vi "Micro-PL v10.6.0.vi"() -> ()   [LabVIEW 2010]
uses:
  drivers/Oxford ITC/ITCAPPS.LLB/ITCSetup.ctl
  drivers/Oxford ITC/ITCSUBS.LLB/ITCIO.ctl
  drivers/Oxford ITC/BUSGEN.LLB/OxfordAddress.ctl
  drivers/Oxford ITC/ITCSUBS.LLB/ITCVersion.ctl
  subvi/NPC3SG/TypeDefs/NPC3SG Live Controls.ctl
  subvi/NPC3SG/TypeDefs/NPC3SG Current Values.ctl
  subvi/NPC3SG/TypeDefs/NPC3SG Set Positions.ctl
  subvi/ITC503/TypeDefs/ITC503 Settings.ctl
  subvi/ITC503/TypeDefs/ITC503 Current Values.ctl
  subvi/iHR550/TypeDefs/iHR Current Values.ctl
  subvi/iHR550/TypeDefs/iHR Settings.ctl
  subvi/Mapping/TypeDefs/Mapping Spectra Params.ctl
  <vilib>/Utility/miscctls.llb/LVBoundsTypeDef.ctl
  subvi/Symphony/TypeDefs/Symphony Area Format.ctl
  <vilib>/Utility/miscctls.llb/LVPointTypeDef.ctl
  subvi/Mapping/TypeDefs/Mapping Input Parameters v10.6.0.ctl
  subvi/Global Variables.vi
  <vilib>/Analysis/NI_AALBase.lvlib
panel:
  out "Spectrum Raw PX":dbl[][](array[numeric])
  out "Image Raw":i32[][](array[numeric])
  in  "Wavelength Recalculate":bool
  out "CCD Error":errorcluster
  out "Firmware":string="V1.20 CCD_4000"
  out "CCD Gain Number":i32[](array[numeric])=[10, 11, 12, 13, 8, 2]
  out "CCD ADC Number":i32[](array[numeric])=[0, 1, 2, 3, 4]
  out "JYCCDLib.IJYCCDReqd":refnum<k7>
  out "Spectrum Raw WL":dbl[][](array[numeric])
  out "Mapping State Storage":bool
  out "Drive Copy Target":bool
  in  "CCD Shutter":bool caption="Shutter:"
  out "Measurement Running":bool
  out "ITC Running":bool
  out "Drive Running":bool
  out "CCD Running":bool
  out "Mono Running":bool
  in  "Exit":bool
  out "Mono Status":bool
  out "Drive Status":bool
  out "CCD Status":bool
  out "ITC Status":bool
  in  "Register":enum32{"Devices", "Acquisition / Mapping"}(tab)
  in  "Snapshot Folder":path=path "C:/Users/WET-KORR/Desktop/Screenshots"
  in  "Camera Name":string="HD USB Camera"
  out "CCD Temp Graph":dbl(graph)=-134.538067
  out "CCD IDs":u16(ring) items=["CCD1"]
  out "ITC Current Values":T1 {"ITC503 Gradient" format="%.2f"; "ITC503 Setpoint" min=-273.0 max=300000.0 step=0.0001 format="%.1f"; "ITC503 I" format="%_1f"; "ITC503 P" format="%_1f"; "ITC503 Temperature" min=0.0 max=1645.0 step=1e-05 format="%.2f"; "ITC503 Heater" min=0.0 max=100.0 step=0.01 scale=0.0..100.0}
  in  "ITC Settings":T2={"ITC503 Set Setpoint"=0.0, "ITC503 Set Auto Heater"=TRUE, "ITC503 Set Auto PID"=TRUE, "P"=0.0, "I"=0.0, "D"=0.0} {"D" min=0.0 max=100.0 step=0.1 format="%.1f"; "I" min=0.0 max=100.0 step=0.1 format="%.1f"; "P" min=0.0 max=100.0 step=0.1 format="%.1f"; "ITC503 Set Setpoint" min=-273.0 max=300000.0 step=0.1 format="%.1f"}
  in  "ITC Configure":bool
  in  "ITC Connect":bool
  in  "ITC Selector":u16(ring) caption="Select Device" items=["ITC503s"]
  out "Drive Current Values":T3 {"Drive Z Position" min=-273.0 max=300000.0 step=0.0001 format="%.3f"; "Drive Y Position" min=-273.0 max=300000.0 step=0.0001 format="%.3f"; "Drive X Position" min=-273.0 max=300000.0 step=0.0001 format="%.3f"}
  in  "Drive Connection":refnum<visa-resource-name>="COM5" caption="COM Port"
  in  "Drive Connect":bool
  out "Mono Timing":u32 caption="Mono"
  out "Drive Timing":u32 caption="Drive"
  out "ITC Timing":u32 caption="ITC"
  out "CCD Timing":u32 caption="CCD"
  in  "Mono Force Init":bool=TRUE caption="iHR550 Force Init"
  in  "Mono Connect":bool
  in  "Mono ID":string(combo)="iHR550" caption="Monochromator ID"
  in  "CCD Gain":u16(ring)=1 caption="Gain Mode" items=["High Light", "Best Dynamic Range", "High Sensitivity"]
  in  "Image Mode":bool caption="Image Mode?"
  in  "CCD Names":u16(ring) caption="CCD ID" items=["Symphony II"]
  in  "CCD Connect":bool
  out "CCD Temperature":dbl caption="Temp. (°C)" min=10.0 max=160.0 step=0.1 format="%.1f"
  out "CCD Pixel X":i32=2048 caption="X Pixels"
  out "CCD Pixel Y":i32=512 caption="Y Pixels"
  out "CCD Data Size":i32=2048 caption="Data Size"
  in  "CCD ADC":u16(ring) caption="ADC Frequency" items=["20 kHz       ", " 1 MHz       ", " 1 MHz Ultra ", "500 kHz Wrap"]
  in  "CCD Configure":bool
  in  "CCD Area":T4={"XStart"=1, "YStart"=1, "XStop"=2048, "YStop"=512, "XBin"=1, "YBin"=1}
  in  "Spectrum Axis":u16(ring)=1 caption="Axis" items=["Pixel", "Wavelength", "Energy"]
  in  "Spectrum Autosave":bool caption="iHR550 Force Init"
  in  "CCD Preview":bool
  in  "CCD Acquire":bool
  in  "Spectrum Settings":T5={"Integration Time"=1.0, "Repetitions"=1, "Mapping Spectra"=TRUE} caption="Mapping Spectra Settings" {"Repetitions" min=1 max=100 step=1; "Integration Time" min=0.1 max=6000.0 step=0.1 format="%.1f"}
  in  "CCD Current Rep.":string="0/0"
  out "Spectrum":cluster{dbl[], dbl[]}[](graph)
  in  "Spectrum Noise":i64 caption="Noise Level"
  in  "Spectrum Load":bool
  in  "Spectrum Save":bool
  out "Image":dbl[][](graph)
  in  "Spectrum Maximize":bool
  in  "Video Show":bool
  in  "Drive GoTo":bool caption="Objective Move Abs."
  in  "Drive New Positions":T6 {"Drive X Set" min=10.0 max=160.0 step=0.1 format="%.3f"; "Drive Z Set" min=10.0 max=160.0 step=0.1 format="%.3f"; "Drive Y Set" min=10.0 max=160.0 step=0.1 format="%.3f"}
  out "Drive Live Current Values":T3 {"Drive Z Position" min=-273.0 max=300000.0 step=0.0001 format="%.3f"; "Drive Y Position" min=-273.0 max=300000.0 step=0.0001 format="%.3f"; "Drive X Position" min=-273.0 max=300000.0 step=0.0001 format="%.3f"}
  in  "Drive Live Controls":T7={"Snapshot"=FALSE, "Move Step"=0.5, "Move Home"=FALSE, "Move Down"=FALSE, "Move Up"=FALSE, "Move Left"=FALSE, "Move Right"=FALSE, "Move Out"=FALSE, "Move In"=FALSE} {"Move Step" min=0.0 max=30.0 step=0.1 format="%.3f"}
  in  "Mapping Start":bool
  in  "Mono Configure":bool
  in  "Mono Settings":T8={"iHR550 Set Exit Mirror"=2, "iHR550 Set Side Exit"=0.0, "iHR550 Set Front Entrance"=0.0, "iHR550 Set Wavelength"=897.9988, "iHR550 Set Grating"=0, "iHR550 Set Grating Switch"=FALSE, "iHR550 Set Wavelength Switch"=FALSE, "iHR550 Set Mirror Switch"=FALSE, "iHR550 Set Slits Switch"=FALSE} {"iHR550 Set Grating" items=["1800"=1, "600"=2, "150"=3]; "iHR550 Set Wavelength" min=0.0 max=1500.0 step=1.0; "iHR550 Set Side Exit" min=0.0 max=2000.0 step=1.0; "iHR550 Set Exit Mirror" items=["Front"=2, "Side"=3]}
  out "Mono Current Values":T9={"iHR 550 Front Entrance"=0.0, "iHR550 Side Exit"=0.0, "iHR550 Wavelength"=897.9988, "iHR550 Exit Mirror"=2, "iHR550 Grating"="1", "Grating Index"=1} {"iHR550 Exit Mirror" items=["EntranceMirror", "ExitMirror", "Front", "Side"]}
  out "ITC Temp Storage":dbl
  out "Runtime":u32
  out "ITC Gradient Time":i64
  out "ITC Read":bool
  out "CCD Read":bool
  out "Mono Read":bool
  out "Drive Read":bool
  out "Spectrum Properties":cluster{"Position":T10, "Plot Area Size":T10}={"Position"={"Width"=36, "Height"=367}, "Plot Area Size"={"Width"=496, "Height"=264}}
  in  "Auto Folder":path caption="Ausgewählter Pfad"
  out "Wavelengths (nm)":dbl[](array[numeric])
  out "iHR550 RefNum":refnum<k7> caption="Mono RefNum out"
  out "ITC Setup":T11={"Description"="", "IO Info"={"Address"={"Com Port"=1, "ISOBUS Address"=1, "GPIB Address"=24, "Communication"=enum."ISOBUS"}, "Version"=enum."ITC503", "Ch 1 dec places"=1, "Ch 2 dec places"=1, "Ch 3 dec places"=1, "Ch1 Name"="", "Ch2 Name"="", "Ch3 Name"=""}}
  # "Correlation Setup"
  # "Active"
  # "Active"
  # "ITC"
  # "iHR"
  # "Drive"
  # "CCD"
  # "Status"
  # "CCD"
  # "ITC"
  # "iHR"
  # "Drive"
  # "Video"
  # "Cryostat"
  # "Drives"
  # "Timing"
  # "Monochromator"
  # "CCD"
  # "CCD"
  # "Acquisition"
  # "Drive Control"
  # "XY"
  # "Z"
  # "Mapping"
  # "Launch the Spectral Mapping VI and Raman Tool Set 2.0 in a new window."
  # "Monochromator"
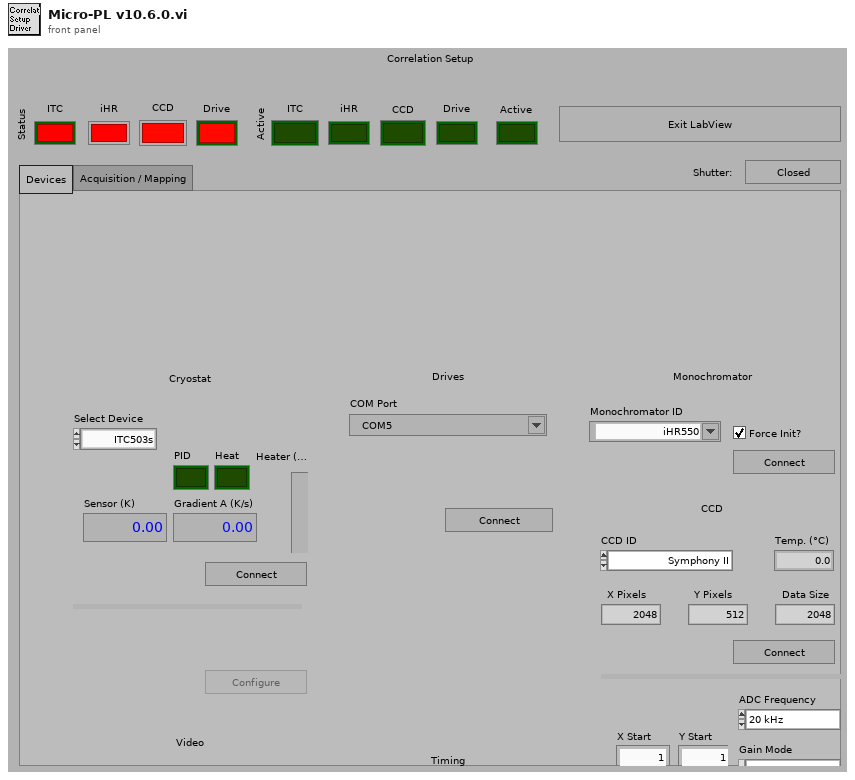
[diagram p1: front panel]
types:
  T1 = typedef "ITC503 Current Values.ctl" = cluster{"ITC503 Heater":dbl, "ITC503 Temperature":dbl, "ITC503 P":dbl, "ITC503 I":dbl, "ITC503 D":dbl, "ITC503 Setpoint":dbl, "ITC503 Gradient":dbl, "ITC503 Heater Auto":bool, "ITC503 PID Auto":bool}
  T2 = typedef "ITC503 Settings.ctl" = cluster{"ITC503 Set Setpoint":dbl, "ITC503 Set Auto Heater":bool, "ITC503 Set Auto PID":bool, "P":dbl, "I":dbl, "D":dbl}
  T3 = typedef "NPC3SG Current Values.ctl" = cluster{"Drive X Position":dbl, "Drive Y Position":dbl, "Drive Z Position":dbl}
  T4 = typedef "Symphony Area Format.ctl" = cluster{"XStart":i32, "YStart":i32, "XStop":i32, "YStop":i32, "XBin":i32, "YBin":i32}
  T5 = typedef "Mapping Spectra Params.ctl" = cluster{"Integration Time":dbl, "Repetitions":u16, "Mapping Spectra":bool}
  T6 = typedef "NPC3SG Set Positions.ctl" = cluster{"Drive X Set":dbl, "Drive Y Set":dbl, "Drive Z Set":dbl}
  T7 = typedef "NPC3SG Live Controls.ctl" = cluster{"Snapshot":bool, "Move Step":dbl, "Move Home":bool, "Move Down":bool, "Move Up":bool, "Move Left":bool, "Move Right":bool, "Move Out":bool, "Move In":bool}
  T8 = typedef "iHR Settings.ctl" = cluster{"iHR550 Set Exit Mirror":u16, "iHR550 Set Side Exit":dbl, "iHR550 Set Front Entrance":dbl, "iHR550 Set Wavelength":dbl, "iHR550 Set Grating":u16, "iHR550 Set Grating Switch":bool, "iHR550 Set Wavelength Switch":bool, "iHR550 Set Mirror Switch":bool, "iHR550 Set Slits Switch":bool}
  T9 = typedef "iHR Current Values.ctl" = cluster{"iHR 550 Front Entrance":dbl, "iHR550 Side Exit":dbl, "iHR550 Wavelength":dbl, "iHR550 Exit Mirror":i32, "iHR550 Grating":string, "Grating Index":i32}
  T10 = typedef "LVBoundsTypeDef.ctl" = cluster{"Width":u32, "Height":u32}
  T11 = typedef "ITCSetup.ctl" = cluster{"Description":string, "IO Info":T12}
  T12 = typedef "ITCIO.ctl" = cluster{"Address":T13, "Version":T14, "Ch 1 dec places":i16, "Ch 2 dec places":i16, "Ch 3 dec places":i16, "Ch1 Name":string, "Ch2 Name":string, "Ch3 Name":string}
  T13 = typedef "OxfordAddress.ctl" = cluster{"Com Port":i32, "ISOBUS Address":i32, "GPIB Address":i16, "Communication":enum16{"RS232", "ISOBUS", "GPIB", "Gateway"}}
  T14 = typedef "ITCVersion.ctl" = enum16{"ITC502", "ITC503", "ITC601"}
  T15 = enum8{"Enabled", "Disabled", "Disabled and Grayed Out"}
  T16 = typedef "LVPointTypeDef.ctl" = cluster{"Horizontal":i16, "Vertical":i16}
  T17 = typedef "Mapping Input Parameters v10.6.0.ctl" = cluster{"Drive Connection Port":refnum<visa-resource-name>, "ITC503 Current Values":T1, "Wavelengths (nm)":dbl[], "Drive Current Values":T3, "iHR Current Values":T9, "Spectra Settings":T5, "CCD3500 Temperature":dbl, "Simulate Drive":bool, "Simulate Spectra":bool, "JYCCDLib.IJYCCDReqd":refnum<k7>, "CCD Area":T4, "CCD Gain":u16, "CCD ADC":u16}
  T18 = cluster{"Intensities":dbl[], "Wavelengths":dbl[]}[]
  T19 = typedef "LVPositionTypeDef.ctl" = cluster{"Left":i32, "Top":i32}
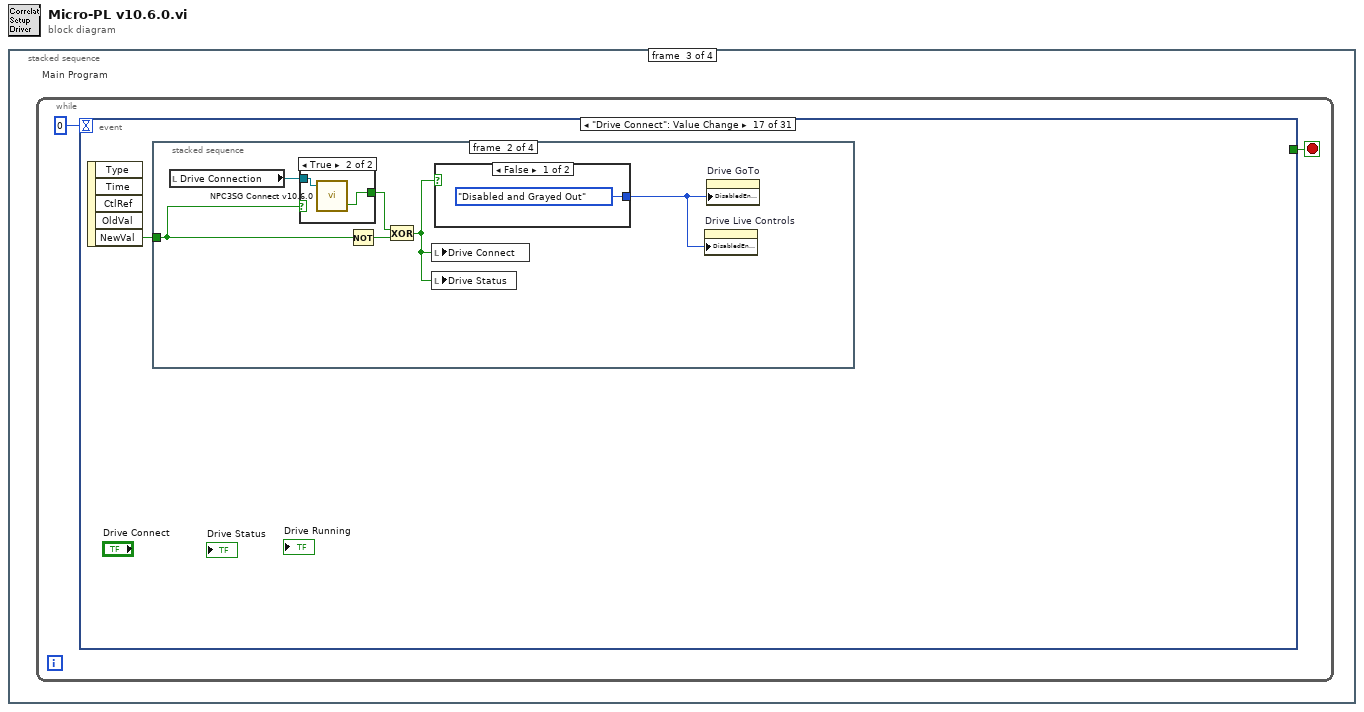
[diagram p0: block diagram]
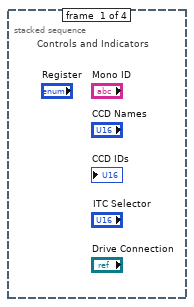
[diagram p2: hidden frame]
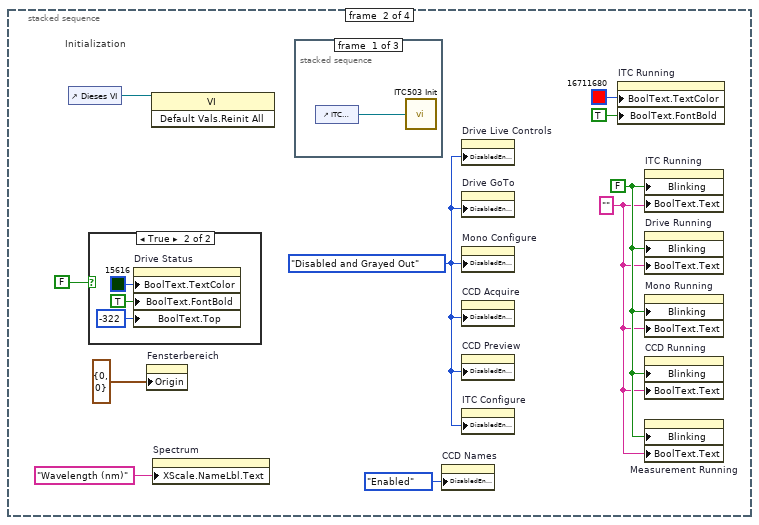
[diagram p3: hidden frame]
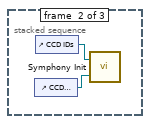
[diagram p4: hidden frame]
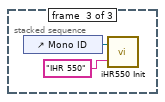
[diagram p5: hidden frame]
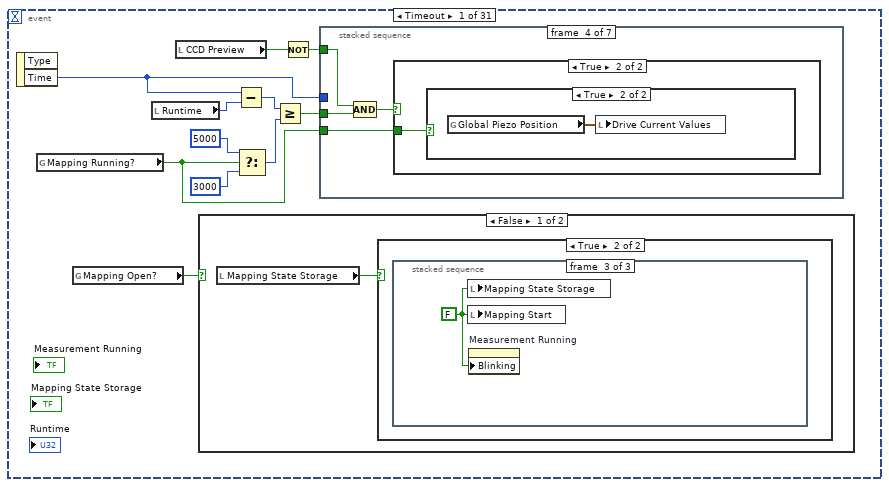
[diagram p7: hidden frame]
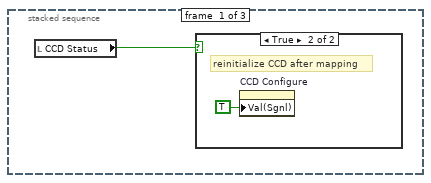
[diagram p9: hidden frame]
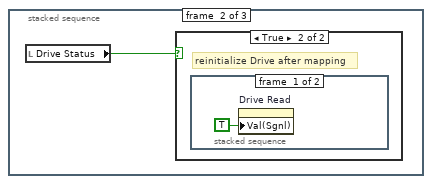
[diagram p11: hidden frame]
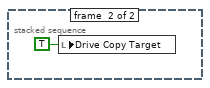
[diagram p13: hidden frame]
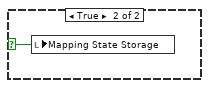
[diagram p14: hidden frame]
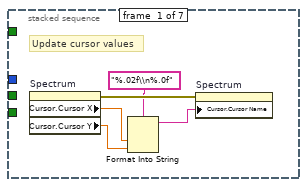
[diagram p15: hidden frame]
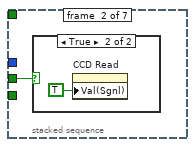
[diagram p16: hidden frame]
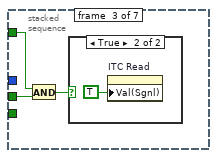
[diagram p18: hidden frame]
diagram:
  n1 = stacked-sequence {
    frame #0 {
      # "Controls and Indicators"
    }
    frame #1 {
      w3 = "" ("Boolean Text.Text")
      w4 = FALSE ("Blinking")
      w7 = T15."Disabled and Grayed Out" ("Deaktiviert")
      # "Initialization"
      n2 = control-ref of="Dieses VI"() -> (w10:refnum<vi>)
      n3 = case shown="True" FALSE {
        frame False {
        }
        frame True {
          n4 = property on="Drive Status" class="Bool (strict)"("BoolText.TextColor"=u32 15616, "BoolText.FontBold"=TRUE ("Boolescher Text.Schriftart:Fett"), "BoolText.Top"=-322 ("Boolescher Text.Position:Oben")) -> ()  [unwired: 2 in, 2 out]
        }
      }
      n5 = property on="Fensterbereich" class="Pane"("Origin"=T16 {"Horizontal"=0, "Vertical"=0}) -> ()  [unwired: 2 in, 2 out]
      n6 = invoke class="VI" method="Default Vals.Reinit All"(reference=w10) -> ()  [unwired: 2 in, 3 out]
      n7 = property on="Spectrum" class="XYGraph (strict)"("XScale.NameLbl.Text"="Wavelength (nm)" ("X Scale.Name Label.Text")) -> ()  [unwired: 2 in, 2 out]
      n8 = stacked-sequence {
        frame #0 {
          n9 = control-ref of="ITC Selector"() -> (w11:refnum<vi>)
          n10 = call "ITC503 Init.vi"("ITC Selector"=w11) -> ()  [unwired: 1 in]
        }
        frame #1 {
          n11 = control-ref of="CCD Names"() -> (w12:refnum<vi>)
          n12 = control-ref of="CCD IDs"() -> (w13:refnum<vi>)
          n13 = call "Symphony Init.vi"("Device Names"=w12, "Device IDs"=w13) -> ()
        }
        frame #2 {
          n14 = control-ref of="Mono ID"() -> (w15:refnum<vi>)
          n15 = call "iHR550 Init.vi"("Mono ID"=w15, "Target ID"="IHR 550") -> ()  [unwired: 1 in]
        }
      }
      n16 = property on="CCD Names" class="Ring (strict)"("DisabledEnum"=T15."Enabled" ("Disabled")) -> ()  [unwired: 2 in, 2 out]
      n17 = property on="Drive Live Controls" class="Clust (strict)"("DisabledEnum"=w7) -> ()  [unwired: 2 in, 2 out]
      n18 = property on="Drive GoTo" class="Bool (strict)"("DisabledEnum"=w7) -> ()  [unwired: 2 in, 2 out]
      n19 = property on="Mono Configure" class="Bool (strict)"("DisabledEnum"=w7) -> ()  [unwired: 2 in, 2 out]
      n20 = property on="CCD Acquire" class="Bool (strict)"("DisabledEnum"=w7) -> ()  [unwired: 2 in, 2 out]
      n21 = property on="CCD Preview" class="Bool (strict)"("DisabledEnum"=w7) -> ()  [unwired: 2 in, 2 out]
      n22 = property on="ITC Configure" class="Bool (strict)"("DisabledEnum"=w7) -> ()  [unwired: 2 in, 2 out]
      n23 = property on="ITC Running" class="Bool (strict)"("BoolText.TextColor"=u32 16711680, "BoolText.FontBold"=TRUE ("Boolean Text.Font:Bold")) -> ()  [unwired: 2 in, 2 out]
      n24 = property on="ITC Running" class="Bool (strict)"("Blinking"=w4, "BoolText.Text"=w3) -> ()  [unwired: 2 in, 2 out]
      n25 = property on="Drive Running" class="Bool (strict)"("Blinking"=w4, "BoolText.Text"=w3) -> ()  [unwired: 2 in, 2 out]
      n26 = property on="Mono Running" class="Bool (strict)"("Blinking"=w4, "BoolText.Text"=w3) -> ()  [unwired: 2 in, 2 out]
      n27 = property on="CCD Running" class="Bool (strict)"("Blinking"=w4, "BoolText.Text"=w3) -> ()  [unwired: 2 in, 2 out]
      n28 = property on="Measurement Running" class="Bool (strict)"("Blinking"=w4, "BoolText.Text"=w3) -> ()  [unwired: 2 in, 2 out]
    }
    frame #2 {
      # "Main Program"
      n29 = while "Main-Program" {
        stop <- w20 stop-if-true
        n30 = event shown="[16] \"Drive Connect\": Value Change" {
          selector: _ -> [_ _ _ _ _ _ _ _ _ _ _ _ _ _ _ _ _ _ _ _ _ _ _ _ _ _ _ _ _ _ _]
          dyn-events: _ -> [_ _ _ _ _ _ _ _ _ _ _ _ _ _ _ _ _ _ _ _ _ _ _ _ _ _ _ _ _ _ _]
          timeout: 0 -> [_ _ _ _ _ _ _ _ _ _ _ _ _ _ _ _ _ _ _ _ _ _ _ _ _ _ _ _ _ _ _]
          tunnel: [_ w69 _ _ _ _ _ _ _ _ _ _ _ _ _ _ _ _ _ _ _ _ _ _ _ _ _ _ _ _ _] -> w20
          event Timeout {
            n31 = event-data() -> ("Time"=w27:u32)  [unwired: 1 in, 1 out]
            n32 = global read "Global Variables.vi" "Mapping Running?"() -> (w22:bool)
            n33 = global read "Global Variables.vi" "Mapping Open?"() -> (w21:bool)
            n34 = local read "Runtime"() -> (w26:u32)
            n35 = local read "CCD Preview"() -> (w29:bool)
            n36 = case shown="False" w21 {
              selector: w21 -> [_ w39]
              frame False {
                n37 = local read "Mapping State Storage"() -> (w32:bool)
                n38 = case shown="True" w32 {
                  frame False {
                  }
                  frame True {
                    n39 = stacked-sequence {
                      frame #0 {
                        n40 = local read "CCD Status"() -> (w33:bool)
                        n41 = case shown="True" w33 {
                          frame False {
                          }
                          frame True {
                            # "reinitialize CCD after mapping"
                            n42 = property on="CCD Configure" class="Bool (strict)"("Val(Sgnl)"=TRUE ("Value (Signaling)")) -> ()  [unwired: 2 in, 2 out]
                          }
                        }
                      }
                      frame #1 {
                        n43 = local read "Drive Status"() -> (w35:bool)
                        n44 = case shown="True" w35 {
                          frame False {
                          }
                          frame True {
                            # "reinitialize Drive after mapping"
                            n45 = stacked-sequence {
                              frame #0 {
                                n46 = property on="Drive Read" class="Bool (strict)"("Val(Sgnl)"=TRUE ("Value (Signaling)")) -> ()  [unwired: 2 in, 2 out]
                              }
                              frame #1 {
                                n47 = local write "Drive Copy Target"(TRUE ("Copy Drive Target")) -> ()
                              }
                            }
                          }
                        }
                      }
                      frame #2 {
                        w38 = FALSE ("Mapping Start")
                        n48 = local write "Mapping State Storage"(w38) -> ()
                        n49 = local write "Mapping Start"(w38) -> ()
                        n50 = property on="Measurement Running" class="Bool (strict)"("Blinking"=w38) -> ()  [unwired: 2 in, 2 out]
                      }
                    }
                  }
                }
              }
              frame True {
                n51 = local write "Mapping State Storage"(w39) -> ()
              }
            }
            n52 = Subtract(x=w27, y=w26) -> (x-y=w30:u32)
            n53 = Select(t=u32 5000 ("y"), s=w22, f=u32 3000 ("y")) -> (s? t:f=w23:u32)
            n54 = Greater Or Equal?(x=w30, y=w23) -> (x >= y?=w31:bool)
            n55 = Not(x=w29) -> (.not. x?=w28:bool)
            n56 = stacked-sequence {
              tunnel: w31 -> [_ w45 w49 w54 w61 _ w66]
              tunnel: w27 -> [_ _ _ _ _ _ w67]
              tunnel: w28 -> [_ _ w48 w53 w60 w63 _]
              tunnel: w22 -> [_ _ _ w51 w58 _ _]
              frame #0 {
                # "Update cursor values"
                n57 = property on="Spectrum" class="XYGraph (strict)"() -> (error out=w44:errorcluster, "Cursor.Cursor X"=w43:dbl, "Cursor.Cursor Y"=w42:dbl)  [unwired: 2 in, 1 out]
                n58 = Format Into String(format string="%.02f\\n%.0f", w43, w42) -> (resulting string=w40:string)  [unwired: 2 in, 1 out]
                n59 = property on="Spectrum" class="XYGraph (strict)"(error in=w44, "Cursor.Cursor Name"=w40) -> ()  [unwired: 1 in, 2 out]
              }
              frame #1 {
                n60 = case shown="True" w45 {
                  frame False {
                  }
                  frame True {
                    n61 = property on="CCD Read" class="Bool (strict)"("Val(Sgnl)"=TRUE ("Value (Signaling)")) -> ()  [unwired: 2 in, 2 out]
                  }
                }
              }
              frame #2 {
                n62 = And(x=w48, y=w49) -> (x .and. y?=w47:bool)
                n63 = case shown="True" w47 {
                  frame False {
                  }
                  frame True {
                    n64 = property on="ITC Read" class="Bool (strict)"("Val(Sgnl)"=TRUE ("Value (Signaling)")) -> ()  [unwired: 2 in, 2 out]
                  }
                }
              }
              frame #3 {
                n65 = Compound Arithmetic op=AND(w53, w54) -> (w52:bool)
                n66 = case shown="True" w52 {
                  tunnel: w51 -> [_ w55]
                  frame False {
                  }
                  frame True {
                    n67 = case shown="True" w55 {
                      frame False {
                        n68 = property on="Drive Read" class="Bool (strict)"("Val(Sgnl)"=TRUE ("Value (Signaling)")) -> ()  [unwired: 2 in, 2 out]
                      }
                      frame True {
                        n69 = global read "Global Variables.vi" "Global Piezo Position"() -> (w57:T3)
                        n70 = local write "Drive Current Values"(w57) -> ()
                      }
                    }
                  }
                }
              }
              frame #4 {
                n71 = Compound Arithmetic op=AND(w60, w61, w58) -> (w59:bool)
                n72 = case shown="True" w59 {
                  frame False {
                  }
                  frame True {
                    n73 = property on="Mono Read" class="Bool (strict)"("Val(Sgnl)"=TRUE ("Value (Signaling)")) -> ()  [unwired: 2 in, 2 out]
                  }
                }
              }
              frame #5 {
                n74 = case shown="False" w63 {
                  frame False {
                    n75 = flat-sequence {
                      frame #0 {
                        w64 = u32 50  # CCD buffer
                        n76 = Wait (ms)(milliseconds to wait=w64) -> ()  [unwired: 1 out]
                      }
                      frame #1 {
                        n77 = property on="CCD Acquire" class="Bool (strict)"("Val(Sgnl)"=TRUE ("Wert (signalisierend)")) -> ()  [unwired: 2 in, 2 out]
                      }
                    }
                  }
                  frame True {
                  }
                }
              }
              frame #6 {
                # "Set runtime counter"
                n78 = case shown="True" w66 {
                  tunnel: w67 -> [_ w68]
                  frame False {
                  }
                  frame True {
                    n79 = local write "Runtime"(w68) -> ()
                  }
                }
              }
            }
          }
          event "Exit": Value Change {
            n80 = event-data() -> ("NewVal"=w69:bool)  [unwired: 1 in, 4 out]
            n81 = stacked-sequence {
              frame #0 {
                n82 = local read "CCD Status"() -> (w70:bool)
                n83 = case shown="True" w70 {
                  frame False {
                  }
                  frame True {
                    n84 = local read "JYCCDLib.IJYCCDReqd"() -> (w71:refnum<k7>)
                    n85 = Close Reference(reference=w71) -> ()  [unwired: 1 in, 1 out]
                  }
                }
              }
              frame #1 {
                n86 = local read "Drive Status"() -> (w72:bool)
                n87 = case shown="True" w72 {
                  frame False {
                  }
                  frame True {
                    n88 = local read "Drive Connection"() -> (w73:refnum<visa-resource-name>)
                    n89 = call "NPC3SG Close.vi"("Drive Visa Name"=w73) -> ()  [unwired: 4 in]
                  }
                }
              }
            }
          }
          event "Mono Connect": Value Change {
            n90 = event-data() -> ("NewVal"=w74:bool)  [unwired: 1 in, 4 out]
            n91 = stacked-sequence {
              tunnel: w74 -> [_ w77 _]
              frame #0 {
                n92 = property on="Mono Running" class="Bool (strict)"("Blinking"=TRUE ("Blinkend")) -> ()  [unwired: 2 in, 2 out]
              }
              frame #1 {
                n93 = case shown="False" w77 {
                  selector: w77 -> [w81 _]
                  tunnel: [w81 w93] -> w76
                  frame False {
                    # "disconnect"
                  }
                  frame True {
                    # "connect"
                    n94 = local read "Mono Force Init"() -> (w91:bool)
                    n95 = control-ref of="iHR550 Set Grating"() -> (w92:refnum<vi>)
                    n96 = local read "Mono ID"() -> (w94:string)
                    n97 = call "iHR550 Connect.vi"("Force\nInitialization"=w91, "Grating Selector"=w92, "Mono ID"=w94) -> ("Initialized"=w93:bool, "iHR550 RefNum"=w90:refnum<k7>)  [unwired: 2 in, 4 out]
                    n98 = local write "iHR550 RefNum"(w90) -> ()
                    n99 = call "iHR550 Read Values v10.5.0.vi"("JYMONOLib.IJYMonoReqd"=w90) -> ("iHR Current Values"=w82:T9)  [unwired: 1 in]
                    n100 = Unbundle By Name(w82) -> ("iHR 550 Front Entrance"=w88:dbl, "iHR550 Side Exit"=w87:dbl, "iHR550 Wavelength"=w86:dbl, "iHR550 Exit Mirror"=w85:i32, "Grating Index"=w83:i32)
                    n101 = local write "Mono Current Values"(w82) -> ()
                    n102 = Bundle By Name(cluster=T8 {"iHR550 Set Exit Mirror"=0, "iHR550 Set Side Exit"=0.0, "iHR550 Set Front Entrance"=0.0, "iHR550 Set Wavelength"=0.0, "iHR550 Set Grating"=0, "iHR550 Set Grating Switch"=FALSE, "iHR550 Set Wavelength Switch"=FALSE, "iHR550 Set Mirror Switch"=FALSE, "iHR550 Set Slits Switch"=FALSE} ("iHR Settings"), "iHR550 Set Front Entrance"=w88, "iHR550 Set Side Exit"=w87, "iHR550 Set Wavelength"=w86, "iHR550 Set Exit Mirror"=w85, "iHR550 Set Grating"=w83) -> (w84:T8)
                    n103 = local write "Mono Settings"(w84) -> ()
                  }
                }
                n104 = case shown="False" w76 {
                  tunnel: [T15."Disabled and Grayed Out" ("Deaktiviert") T15."Enabled" ("Deaktiviert")] -> w78
                  frame False {
                  }
                  frame True {
                  }
                }
                n105 = local write "Mono Connect"(w76) -> ()
                n106 = local write "Mono Status"(w76) -> ()
                n107 = property on="Mono Configure" class="Bool (strict)"("DisabledEnum"=w78) -> ()  [unwired: 2 in, 2 out]
              }
              frame #2 {
                w96 = TRUE ("Wert (signalisierend)")
                w95 = FALSE ("Blinkend")
                n108 = local write "Mono Force Init"(w95) -> ()
                n109 = property on="Mono Running" class="Bool (strict)"("Blinking"=w95) -> ()  [unwired: 2 in, 2 out]
                n110 = property on="Mono Read" class="Bool (strict)"("Val(Sgnl)"=w96) -> ()  [unwired: 2 in, 2 out]
                n111 = property on="Wavelength Recalculate" class="Bool (strict)"("Val(Sgnl)"=w96) -> ()  [unwired: 2 in, 2 out]
              }
            }
          }
          event "Mono Read": Value Change {
            n112 = event-data() -> ("NewVal"=w100:bool)  [unwired: 1 in, 4 out]
            n113 = local read "Mono Status"() -> (w99:bool)
            n114 = And(x=w99, y=w100) -> (x .and. y?=w98:bool)
            n115 = case shown="False" w98 {
              tunnel: [u32 0 w102] -> w97
              frame False {
              }
              frame True {
                n116 = stacked-sequence {
                  seq-local: [w103 _ _] -> [_ _ w106]
                  tunnel: [_ _ w107] -> w102
                  frame #0 {
                    n117 = Tick Count (ms)() -> (millisecond timer value=w103:u32)
                  }
                  frame #1 {
                    n118 = local read "iHR550 RefNum"() -> (w105:refnum<k7>)
                    n119 = call "iHR550 Read Values v10.5.0.vi"("JYMONOLib.IJYMonoReqd"=w105) -> ("iHR Current Values"=w104:T9)  [unwired: 1 in]
                    n120 = local write "Mono Current Values"(w104) -> ()
                    n121 = global write "Global Variables.vi" "Global iHR Values"(w104) -> ()
                  }
                  frame #2 {
                    n122 = Tick Count (ms)() -> (millisecond timer value=w108:u32)
                    n123 = Subtract(x=w108, y=w106) -> (x-y=w107:u32)
                  }
                }
              }
            }
            "Mono Timing" <- w97
          }
          event "Mono Configure": Value Change {
            n124 = event-data() -> ("NewVal"=w109:bool)  [unwired: 1 in, 4 out]
            n125 = stacked-sequence {
              tunnel: w109 -> [_ w111 _]
              frame #0 {
                n126 = property on="Mono Running" class="Bool (strict)"("Blinking"=TRUE ("Blinkend")) -> ()  [unwired: 2 in, 2 out]
              }
              frame #1 {
                n127 = local read "Mono Status"() -> (w113:bool)
                n128 = And(x=w113, y=w111) -> (x .and. y?=w112:bool)
                n129 = case shown="True" w112 {
                  frame False {
                  }
                  frame True {
                    n130 = stacked-sequence {
                      frame #0 {
                        w117 = u16 2 items=["Front"=2, "Side"=3] ("Entrance Mirror")
                        n131 = local read "iHR550 RefNum"() -> (w114:refnum<k7>)
                        n132 = local read "Mono Settings"() -> (w115:T8)
                        n133 = call "iHR550 Set Values v10.5.0.vi"("Refnum out"=w114, "Entrance Mirror"=w117, "Target\nSide Entrance"=0.0 ("Target\nSide Entrance"), "iHR Settings"=w115) -> ()  [unwired: 11 in, 1 out]
                      }
                      frame #1 {
                        n134 = property on="Mono Read" class="Bool (strict)"("Val(Sgnl)"=TRUE ("Value (Signaling)")) -> ()  [unwired: 2 in, 2 out]
                      }
                      frame #2 {
                        n135 = property on="Wavelength Recalculate" class="Bool (strict)"("Val(Sgnl)"=TRUE ("Value (Signaling)")) -> ()  [unwired: 2 in, 2 out]
                      }
                    }
                  }
                }
              }
              frame #2 {
                w121 = FALSE ("Blinkend")
                n136 = property on="Mono Read" class="Bool (strict)"("Val(Sgnl)"=TRUE ("Wert (signalisierend)")) -> ()  [unwired: 2 in, 2 out]
                n137 = property on="Mono Running" class="Bool (strict)"("Blinking"=w121) -> ()  [unwired: 2 in, 2 out]
                n138 = local write "Mono Configure"(w121) -> ()
              }
            }
          }
          event "CCD Connect": Value Change {
            n139 = event-data() -> ("NewVal"=w122:bool)  [unwired: 1 in, 4 out]
            n140 = stacked-sequence {
              tunnel: w122 -> [_ w126 _]
              frame #0 {
                n141 = local read "CCD Names"() -> (w123:u16)
                n142 = property on="CCD Running" class="Bool (strict)"("Blinking"=TRUE ("Blinkend")) -> ()  [unwired: 2 in, 2 out]
                n143 = local write "CCD IDs"(w123) -> ()
              }
              frame #1 {
                n144 = case shown="False" w126 {
                  selector: w126 -> [w135 _]
                  tunnel: [w135 w144] -> w128
                  frame False {
                    # "disconnect"
                    n145 = local read "JYCCDLib.IJYCCDReqd"() -> (w134:refnum<k7>)
                    n146 = local read "CCD Error"() -> (w133:errorcluster)
                    n147 = Close Reference(reference=w134, error in (no error)=w133) -> ()  [unwired: 1 out]
                  }
                  frame True {
                    # "connect"
                    n148 = local read "CCD IDs"() -> (w149:u16)
                    n149 = property on="CCD IDs" class="Ring (strict)"() -> ("Chaînes []"=w148:string[])  [unwired: 2 in, 2 out]
                    n150 = Index Array(array=w148, index=w149) -> (element=w150:string)
                    n151 = call "Initialize CCD.vi"("Unique id:"=w150) -> ("activeYPixels"=w137:i32, "JYCCDLib.IJYCCDReqd"=w151:refnum<k7>, "activeXPixels"=w139:i32, "sortie d'erreur"=w152:errorcluster, "FirmwareVersion"=→"Firmware":string)  [unwired: 3 out]
                    "CCD Pixel X" <- w139
                    "CCD Pixel Y" <- w137
                    n152 = call "Trigger - Disable.vi"("Error In"=w152, "JYCCDLib.IJYCCDReqd"=w151) -> ("Error Out"=w146:errorcluster, "JYCCDLib.IJYCCDReqd"=w157:refnum<k7>)  [unwired: 4 out]
                    n153 = local read "CCD Area"() -> (w143:T4)
                    n154 = Bundle By Name(cluster=w143, "XStart"=1, "XStop"=w139, "YStart"=1, "YStop"=w137, "XBin"=1, "YBin"=1) -> (w142:T4)
                    n155 = local write "CCD Error"(w146) -> ()
                    n156 = call "Init ADC & Gain.vi"("JYCCDLib.IJYCCDReqd"=w157, "input error"=w146) -> ("ADC Number"=w153:i32[], "ADC description"=w155:string[], "Gain Number"=w154:i32[], "Gain description"=w156:string[])
                    n157 = local write "JYCCDLib.IJYCCDReqd"(w157) -> ()
                    n158 = local write "CCD Area"(w142) -> ()
                    n159 = local write "CCD ADC Number"(w153) -> ()
                    n160 = local write "CCD Gain Number"(w154) -> ()
                    n161 = property on="CCD ADC" class="Ring (strict)"("Chaînes []"=w155) -> ()  [unwired: 2 in, 2 out]
                    n162 = property on="CCD Gain" class="Ring (strict)"("Chaînes []"=w156) -> ()  [unwired: 2 in, 2 out]
                    n163 = call <vilib>:"Simple Error Handler.vi"("error in (no error)"=w146) -> ("error?"=w145:bool)  [unwired: 4 in, 4 out]
                    n164 = Not(x=w145) -> (.not. x?=w144:bool)
                  }
                }
                n165 = case shown="False" w128 {
                  tunnel: [T15."Disabled and Grayed Out" ("Deaktiviert") T15."Enabled" ("Deaktiviert")] -> w127
                  tunnel: [T15."Enabled" ("Deaktiviert") T15."Disabled and Grayed Out" ("Deaktiviert")] -> w125
                  frame False {
                  }
                  frame True {
                  }
                }
                n166 = property on="CCD Status" class="Bool (strict)"("BoolText.Visible"=w128) -> ()  [unwired: 2 in, 2 out]
                n167 = local write "CCD Connect"(w128) -> ()
                n168 = local write "CCD Status"(w128) -> ()
                n169 = property on="CCD Acquire" class="Bool (strict)"("DisabledEnum"=w127) -> ()  [unwired: 2 in, 2 out]
                n170 = property on="CCD Preview" class="Bool (strict)"("DisabledEnum"=w127) -> ()  [unwired: 2 in, 2 out]
                n171 = property on="CCD Names" class="Ring (strict)"("Désactivé"=w125) -> ()  [unwired: 2 in, 2 out]
                n172 = property on="CCD IDs" class="Ring (strict)"("Désactivé"=w125) -> ()  [unwired: 2 in, 2 out]
              }
              frame #2 {
                w158 = TRUE ("Wert (signalisierend)")
                n173 = property on="CCD Configure" class="Bool (strict)"("Val(Sgnl)"=w158) -> (error out=w159:errorcluster)  [unwired: 2 in, 1 out]
                n174 = property on="CCD Running" class="Bool (strict)"("Blinking"=FALSE ("Blinkend")) -> ()  [unwired: 2 in, 2 out]
                n175 = property on="CCD Read" class="Bool (strict)"(error in=w159, "Val(Sgnl)"=w158) -> ()  [unwired: 1 in, 2 out]
              }
            }
          }
          event "CCD Read": Value Change {
            n176 = event-data() -> ("NewVal"=w164:bool)  [unwired: 1 in, 4 out]
            n177 = local read "CCD Status"() -> (w163:bool)
            n178 = And(x=w163, y=w164) -> (x .and. y?=w162:bool)
            n179 = case shown="True" w162 {
              tunnel: [u32 0 w166] -> w161
              frame False {
              }
              frame True {
                n180 = stacked-sequence {
                  seq-local: [_ w168 _ _] -> [_ _ w173 _]
                  seq-local: [w167 _ _ _] -> [_ _ _ w184]
                  tunnel: [_ _ _ w185] -> w166
                  frame #0 {
                    n181 = Tick Count (ms)() -> (millisecond timer value=w167:u32)
                  }
                  frame #1 {
                    w169 = u16 0 items=["° Celsius", "Kelvin", "° Farenheit"] ("units")
                    n182 = local read "JYCCDLib.IJYCCDReqd"() -> (w172:refnum<k7>)
                    n183 = local read "CCD Error"() -> (w170:errorcluster)
                    n184 = call "read temperature.vi"("entrée d'erreur (pas d'erreur)"=w170, "units"=w169, "JYCCDLib.IJYCCDReqd"=w172) -> ("error out"=w171:errorcluster, "Current Temperature"=w168:dbl)
                    n185 = local write "CCD Temp Graph"(w168) -> ()
                    n186 = local write "CCD Error"(w171) -> ()
                    n187 = local write "CCD Temperature"(w168) -> ()
                  }
                  frame #2 {
                    n188 = Greater?(x=w173, y=-130.0) -> (0:w174:bool)
                    n189 = case shown="False" w174 {
                      selector: w174 -> [w181 w183]
                      tunnel: [cluster{u32, u32}[] [{16713728, 16713728}, {6618880, 6618880}] ("Farben [4]") cluster{u32, u32}[] [{16713728, 16713728}] ("Farben [4]")] -> w175
                      tunnel: [w181 w183] -> w177
                      frame False {
                      }
                      frame True {
                      }
                    }
                    n190 = Number To Fractional String(number=w173, precision (6)=i16 1 ("Genauigkeit (6)")) -> (F-format string=w176:string)  [unwired: 2 in]
                    n191 = global write "Global Variables.vi" "Global CCD Temperature (C)"(w173) -> ()
                    n192 = property on="CCD Status" class="Bool (strict)"("Blinking"=w177, "BoolText.Text"=w176, "Colors [4]"=w175) -> ()  [unwired: 2 in, 2 out]
                  }
                  frame #3 {
                    n193 = Tick Count (ms)() -> (millisecond timer value=w186:u32)
                    n194 = Subtract(x=w186, y=w184) -> (x-y=w185:u32)
                  }
                }
              }
            }
            "CCD Timing" <- w161
          }
          event "CCD Configure": Value Change {
            n195 = event-data() -> ("NewVal"=w188:bool)  [unwired: 1 in, 4 out]
            n196 = local read "CCD Status"() -> (w189:bool)
            n197 = And(x=w189, y=w188) -> (x .and. y?=w187:bool)
            n198 = case shown="True" w187 {
              frame False {
              }
              frame True {
                n199 = stacked-sequence {
                  frame #0 {
                    n200 = local read "Spectrum Settings"() -> (w194:T5)
                    n201 = local read "CCD Gain Number"() -> (w203:i32[])
                    n202 = local read "CCD ADC Number"() -> (w201:i32[])
                    n203 = local read "JYCCDLib.IJYCCDReqd"() -> (w192:refnum<k7>)
                    n204 = local read "CCD ADC"() -> (w200:u16)
                    n205 = local read "CCD Gain"() -> (w202:u16)
                    n206 = Unbundle By Name(w194) -> ("Integration Time"=w193:dbl)
                    n207 = local read "Image Mode"() -> (w197:bool)
                    n208 = local read "CCD Error"() -> (w196:errorcluster)
                    n209 = local read "CCD Area"() -> (w191:T4)
                    n210 = Index Array(array=w201, index=w200) -> (element=w199:i32)
                    n211 = Index Array(array=w203, index=w202) -> (element=w198:i32)
                    n212 = call "Symphony Setup.vi"("JYCCDLib.IJYCCDReqd"=w192, "ADC"=w199, "Image Mode"=w197, "Integration (s)"=w193, "Symphony Area Format"=w191, "Error Input"=w196, "Gain"=w198) -> ("DataSize"=w190:i32, "Error Output"=w195:errorcluster)  [unwired: 7 in]
                    n213 = local write "CCD Error"(w195) -> ()
                    n214 = local write "CCD Data Size"(w190) -> ()
                  }
                  frame #1 {
                    n215 = property on="Wavelength Recalculate" class="Bool (strict)"("Val(Sgnl)"=TRUE ("Value (Signaling)")) -> ()  [unwired: 2 in, 2 out]
                    n216 = local write "CCD Configure"(FALSE ("CCD Configure")) -> ()
                    n217 = local read "Image Mode"() -> (w205:bool)
                    n218 = Not(x=w205) -> (.not. x?=w204:bool)
                    n219 = property on="Spectrum" class="XYGraph (strict)"("Visible"=w204) -> ()  [unwired: 2 in, 2 out]
                    n220 = property on="Spectrum Load" class="Bool (strict)"("Visible"=w204) -> ()  [unwired: 2 in, 2 out]
                    n221 = property on="Spectrum Noise" class="DigNum (strict)"("Visible"=w204) -> ()  [unwired: 2 in, 2 out]
                    n222 = property on="CCD Current Rep." class="Str"("Visible"=w204) -> ()  [unwired: 2 in, 2 out]
                    n223 = property on="Image" class="IntGraph (strict)"("Visible"=w205) -> ()  [unwired: 2 in, 2 out]
                  }
                }
              }
            }
          }
          event Value Change {
            n224 = event-data() -> ()  [unwired: 1 in, 5 out]
            n225 = stacked-sequence {
              frame #0 {
                w221 = 1 ("y")
                n226 = local read "CCD Area"() -> (w219:T4)
                n227 = Unbundle By Name(w219) -> ("XBin"=w215:i32, "YBin"=w220:i32)
                n228 = Logarithm Base 2(1:w220) -> (0:w216:dbl)
                n229 = Logarithm Base 2(1:w215) -> (0:w212:dbl)
                n230 = Quotient & Remainder(x=w216, y=w221) -> (x-y*floor(x/y)=w217:dbl, floor(x/y)=w218:dbl)
                n231 = Quotient & Remainder(x=w212, y=w221) -> (x-y*floor(x/y)=w213:dbl, floor(x/y)=w214:dbl)
                n232 = Not Equal To 0?(x=w217) -> (x != 0?=w211:bool)
                n233 = Not Equal To 0?(x=w213) -> (x != 0?=w210:bool)
                n234 = Or(x=w210, y=w211) -> (x .or. y?=w209:bool)
                n235 = case shown="True" w211 {
                  tunnel: w218 -> [_ w226]
                  tunnel: w219 -> [_ w224]
                  frame False {
                  }
                  frame True {
                    n236 = Power Of 2(x=w226) -> (2^x=w225:dbl)
                    n237 = Bundle By Name(cluster=w224, "YBin"=w225) -> (w223:T4)
                    n238 = local write "CCD Area"(w223) -> ()
                  }
                }
                n239 = case shown="True" w210 {
                  tunnel: w214 -> [_ w230]
                  tunnel: w219 -> [_ w228]
                  frame False {
                  }
                  frame True {
                    n240 = Power Of 2(x=w230) -> (2^x=w229:dbl)
                    n241 = Bundle By Name(cluster=w228, "XBin"=w229) -> (w227:T4)
                    n242 = local write "CCD Area"(w227) -> ()
                  }
                }
                n243 = case shown="True" w209 {
                  tunnel: "Binning factor has been adjusted  (must be an exponent of 2)." ("message") -> [_ w222]
                  frame False {
                  }
                  frame True {
                    n244 = One Button Dialog(message=w222) -> ()  [unwired: 1 in, 1 out]
                  }
                }
              }
              frame #1 {
                w249 = "Could not adjust CCD area to fit binning size!" ("message")
                w250 = "CCD area has been adjusted to fit binning size." ("message")
                n245 = local read "CCD Area"() -> (w231:T4)
                n246 = Unbundle By Name(w231) -> ("XStop"=w238:i32, "XStart"=w239:i32, "XBin"=w236:i32)
                n247 = Unbundle By Name(w231) -> ("YStop"=w243:i32, "YStart"=w244:i32, "YBin"=w248:i32)
                n248 = Subtract(x=w238, y=w239) -> (x-y=w232:i32)
                n249 = Subtract(x=w243, y=w244) -> (x-y=w241:i32)
                n250 = Increment(x=w232) -> (x+1=w237:i32)
                n251 = Increment(x=w241) -> (x+1=w245:i32)
                n252 = Quotient & Remainder(x=w237, y=w236) -> (x-y*floor(x/y)=w233:i32, floor(x/y)=w235:i32)
                n253 = Quotient & Remainder(x=w245, y=w248) -> (x-y*floor(x/y)=w242:i32, floor(x/y)=w247:i32)
                n254 = Not Equal To 0?(x=w233) -> (x != 0?=w234:bool)
                n255 = Not Equal To 0?(x=w242) -> (x != 0?=w246:bool)
                n256 = case shown="True" w246 {
                  tunnel: w243 -> [_ w268]
                  tunnel: w244 -> [_ w267]
                  tunnel: w245 -> [_ w266]
                  tunnel: w247 -> [_ w265]
                  tunnel: w248 -> [_ w264]
                  tunnel: w249 -> [_ w258]
                  tunnel: w250 -> [_ w259]
                  tunnel: w231 -> [_ w263]
                  tunnel: ["" ("message") w260] -> w252
                  frame False {
                  }
                  frame True {
                    n257 = Multiply(x=w265, y=w264) -> (x*y=w270:i32)
                    n258 = Subtract(x=w266, y=w270) -> (x-y=w269:i32)
                    n259 = Add(x=w267, y=w269) -> (x+y=w262:i32)
                    n260 = Greater?(x=w268, y=w262) -> (0:w261:bool)
                    n261 = case shown="True" w261 {
                      tunnel: w263 -> [_ w275]
                      tunnel: w262 -> [_ w274]
                      tunnel: [w271 w272] -> w260
                      tunnel: w259 -> [_ w272]
                      tunnel: w258 -> [w271 _]
                      frame False {
                      }
                      frame True {
                        n262 = Bundle By Name(cluster=w275, "YStart"=w274) -> (w273:T4)
                        n263 = local write "CCD Area"(w273) -> ()
                      }
                    }
                  }
                }
                n264 = case shown="True" w234 {
                  tunnel: w235 -> [_ w290]
                  tunnel: w236 -> [_ w289]
                  tunnel: w237 -> [_ w283]
                  tunnel: w238 -> [_ w286]
                  tunnel: w239 -> [_ w284]
                  tunnel: w231 -> [_ w282]
                  tunnel: ["" ("message") w280] -> w253
                  tunnel: w250 -> [_ w279]
                  tunnel: w249 -> [_ w278]
                  frame False {
                  }
                  frame True {
                    n265 = Multiply(x=w290, y=w289) -> (x*y=w288:i32)
                    n266 = Subtract(x=w283, y=w288) -> (x-y=w285:i32)
                    n267 = Add(x=w284, y=w285) -> (x+y=w281:i32)
                    n268 = Greater?(x=w286, y=w281) -> (0:w287:bool)
                    n269 = case shown="True" w287 {
                      tunnel: w282 -> [_ w295]
                      tunnel: w281 -> [_ w293]
                      tunnel: [w291 w292] -> w280
                      tunnel: w279 -> [_ w292]
                      tunnel: w278 -> [w291 _]
                      frame False {
                      }
                      frame True {
                        n270 = Bundle By Name(cluster=w295, "XStart"=w293) -> (w294:T4)
                        n271 = local write "CCD Area"(w294) -> ()
                      }
                    }
                  }
                }
                n272 = Empty String/Path?(string/path=w253) -> (empty?=w251:bool)
                n273 = case shown="False" w251 {
                  tunnel: [w255 w256] -> w254
                  tunnel: w252 -> [_ w256]
                  tunnel: w253 -> [w255 _]
                  frame False {
                  }
                  frame True {
                  }
                }
                n274 = Empty String/Path?(string/path=w254) -> (empty?=w240:bool)
                n275 = case shown="False" w240 {
                  tunnel: w254 -> [w276 _]
                  frame False {
                    n276 = One Button Dialog(message=w276) -> ()  [unwired: 1 in, 1 out]
                  }
                  frame True {
                  }
                }
              }
            }
          }
          event "Image Mode": Value Change {
            # "For Symphony (II), ADC0 is\n20 kHz and ADC1 is 1 MHz.\nThis couples the selected  ADC\nto the imaging mode selection."
            n277 = event-data() -> ("NewVal"=w299:bool)  [unwired: 1 in, 4 out]
            n278 = Select(t=i8 1, s=w299, f=i8 0) -> (s? t:f=w298:i8)
            n279 = property on="CCD ADC" class="Ring (strict)"("Val(Sgnl)"=w298) -> ()  [unwired: 2 in, 2 out]
          }
          event "CCD Shutter": Value Change {
            n280 = event-data() -> ("NewVal"=w300:bool)  [unwired: 1 in, 4 out]
            n281 = local read "CCD Status"() -> (w301:bool)
            n282 = case shown="False" w301 {
              tunnel: w300 -> [_ w303]
              frame False {
              }
              frame True {
                n283 = local read "JYCCDLib.IJYCCDReqd"() -> (w305:refnum<k7>)
                n284 = local read "CCD Error"() -> (w304:errorcluster)
                n285 = call "Shutter Control.vi"("input error"=w304, "Shutter"=w303, "JYCCDLib.IJYCCDReqd"=w305) -> ("error out"=w306:errorcluster)  [unwired: 1 out]
                n286 = call <vilib>:"Simple Error Handler.vi"("error in (no error)"=w306) -> ("error?"=w302:bool)  [unwired: 4 in, 4 out]
                n287 = local write "CCD Error"(w306) -> ()
                n288 = case shown="True" w302 {
                  tunnel: w303 -> [_ w307]
                  frame False {
                  }
                  frame True {
                    n289 = Not(x=w307) -> (.not. x?=w308:bool)
                    n290 = local write "CCD Shutter"(w308) -> ()
                  }
                }
              }
            }
          }
          event "CCD Acquire": Value Change {
            n291 = event-data() -> ("NewVal"=w309:bool)  [unwired: 1 in, 4 out]
            n292 = case shown="False" w309 {
              frame False {
              }
              frame True {
                n293 = stacked-sequence {
                  frame #0 {
                    n294 = local read "JYCCDLib.IJYCCDReqd"() -> (w310:refnum<k7>)
                    n295 = local read "Image Mode"() -> (w314:bool)
                    n296 = local read "CCD Error"() -> (w311:errorcluster)
                    n297 = control-ref of="CCD Acquire"() -> (w312:refnum<vi>)
                    n298 = control-ref of="CCD Running"() -> (w313:refnum<vi>)
                    n299 = case shown="False" w314 {
                      tunnel: w313 -> [w318 w369]
                      tunnel: w312 -> [w317 w368]
                      tunnel: w311 -> [w316 w370]
                      tunnel: w310 -> [w315 w371]
                      frame False {
                        n300 = local read "CCD Preview"() -> (w319:bool)
                        n301 = local read "Spectrum Settings"() -> (w320:T5)
                        n302 = Unbundle By Name(w320) -> ("Repetitions"=w323:u16)
                        n303 = Select(t=i8 1, s=w319, f=w323) -> (s? t:f=w322:u16)
                        n304 = for {
                          N: w322 -> [w352]
                          tunnel: w315 -> [w344]
                          shift-right: [w357] -> _
                          shift-left: u16[][] [] -> [w358]
                          tunnel: w318 -> [w339]
                          tunnel: w317 -> [w338]
                          tunnel: w316 -> [w337]
                          i -> [w353]
                          stop <- w356 continue-if-true
                          w332 = u16 0 items=["Pixel", "Wavelength", "Energy"] ("Spectrum Axis")
                          w335 = u16 2 items=["Pixel", "Wavelength", "Energy"] ("Spectrum Axis")
                          n305 = Number To Decimal String(number=w352) -> (decimal integer string=w351:string)  [unwired: 1 in]
                          n306 = Increment(x=w353) -> (x+1=w349:i32)
                          n307 = call "Symphony Acquire Spectrum.vi"("Acquire"=w338, "Running"=w339, "Error In"=w337, "ShutterOpen"=TRUE, "JYCCDLib.IJYCCDReqd"=w344) -> ("Acq Time(ms)"=w336:u32, "Raw Data"=w342:i32[][])  [unwired: 5 in]
                          n308 = Number To Decimal String(number=w349) -> (decimal integer string=w350:string)  [unwired: 1 in]
                          n309 = local write "CCD Timing"(w336) -> ()
                          n310 = Index Array(array=w342, index (row)=0) -> (element=w340:i32[])  [unwired: 1 in]
                          n311 = Concatenate Strings(w350, "/" ("string"), w351) -> (w355:string)
                          n312 = local write "CCD Current Rep."(w355) -> ()
                          n313 = Build Array (concatenate)(w340, w358) -> (w357:i32[][])
                          n314 = local read "Wavelengths (nm)"() -> (w330:dbl[])
                          n315 = local read "Spectrum Axis"() -> (w333:u16)
                          n316 = local read "CCD Area"() -> (w329:T4)
                          n317 = call "Symphony Average Spectra.vi"("Repetitions"=w349, "Raw Spectra"=w357) -> ("Raw Spectrum"=w328:dbl[])
                          n318 = Not Equal?(x=w332, y=w333) -> (x != y?=w331:bool)
                          n319 = Equal?(x=w333, y=w335) -> (x = y?=w334:bool)
                          n320 = call "Spectrum Merge Pixels v10.5.0.vi"("CCD Area Format"=w329, "Raw Spectrum"=w328) -> ("Spectrum-Array"=w326:dbl[][])  [unwired: 1 out]
                          n321 = call "Spectrum Merge Wavelengths v10.5.0.vi"("Wavelengths (nm)"=w330, "Raw Spectrum"=w328) -> ("Spectrum-Array"=w325:dbl[][])  [unwired: 1 out]
                          n322 = local read "Spectrum Noise"() -> (w348:i64)
                          n323 = case shown="False" w331 {
                            tunnel: [w359 w360] -> w327
                            tunnel: w325 -> [_ w360]
                            tunnel: w326 -> [w359 _]
                            frame False {
                            }
                            frame True {
                            }
                          }
                          n324 = call "Spectrum Noise Subtraction v10.5.0.vi"("Spectrum Noise"=w348, "Spectrum-Array In"=w327) -> ("Spectrum-Array Out"=w347:dbl[][], "Spectrum-Cluster"=w345:T18)
                          n325 = local write "Spectrum Raw PX"(w326) -> ()
                          n326 = local write "Spectrum Raw WL"(w325) -> ()
                          n327 = case shown="False" w334 {
                            tunnel: w347 -> [_ w363]
                            tunnel: [w361 w362] -> w346
                            tunnel: w345 -> [w361 _]
                            frame False {
                            }
                            frame True {
                              n328 = call "Spectrum Jacobian Transformation v10.5.0.vi"("Spectrum-Array In"=w363) -> ("Spectrum-Cluster"=w362:T18)  [unwired: 1 in, 1 out]
                            }
                          }
                          n329 = local read "CCD Acquire"() -> (w356:bool)
                          n330 = local write "Spectrum"(w346) -> ()
                        }
                      }
                      frame True {
                        n331 = call "Symphony Acquire Image.vi"("Acquire"=w368, "Running"=w369, "Error In"=w370, "ShutterOpen"=TRUE, "JYCCDLib.IJYCCDReqd"=w371) -> ("Acq Time(ms)"=w364:u32, "Raw Data"=w367:i32[][][])  [unwired: 5 in]
                        n332 = local write "CCD Timing"(w364) -> ()
                        n333 = Index Array(array=w367, index (dim 0)=0 ("index (row)")) -> (element=w365:i32[][])  [unwired: 2 in]
                        n334 = local write "Image Raw"(w365) -> ()
                        n335 = local write "Image"(w365) -> ()
                      }
                    }
                  }
                  frame #1 {
                    n336 = local write "CCD Acquire"(FALSE ("Blinkend")) -> ()
                    n337 = local write "CCD Current Rep."("0/0" ("CCD3000 Current Rep.")) -> ()
                    n338 = local read "Spectrum Autosave"() -> (w375:bool)
                    n339 = case shown="False" w375 {
                      frame False {
                      }
                      frame True {
                        n340 = property on="Spectrum Save" class="Bool (strict)"("Val(Sgnl)"=TRUE ("Value (Signaling)")) -> ()  [unwired: 2 in, 2 out]
                      }
                    }
                  }
                }
              }
            }
          }
          event "CCD Preview": Value Change {
            n341 = event-data() -> ("NewVal"=w377:bool)  [unwired: 1 in, 4 out]
            n342 = case shown="False" w377 {
              frame False {
              }
              frame True {
                n343 = property on="CCD Acquire" class="Bool (strict)"("Val(Sgnl)"=TRUE ("Wert (signalisierend)")) -> ()  [unwired: 2 in, 2 out]
              }
            }
          }
          event "ITC Connect": Value Change {
            n344 = event-data() -> ("NewVal"=w379:bool)  [unwired: 1 in, 4 out]
            n345 = stacked-sequence {
              tunnel: w379 -> [_ w381 _]
              frame #0 {
                n346 = property on="ITC Running" class="Bool (strict)"("Blinking"=TRUE ("Blinkend")) -> ()  [unwired: 2 in, 2 out]
              }
              frame #1 {
                n347 = case shown="False" w381 {
                  selector: w381 -> [w386 _]
                  tunnel: [w386 w393] -> w383
                  frame False {
                    # "disconnect"
                    n348 = control-ref of="ITC Running"() -> (w387:refnum<vi>)
                    n349 = property class="Bool (strict)"(reference=w387, "Blinking"=w386, "Value"=w386) -> ()  [unwired: 1 in, 2 out]
                  }
                  frame True {
                    # "connect"
                    n350 = local read "ITC Selector"() -> (w394:u16)
                    n351 = call "ITC503 Connect.vi"("ITC Selector"=w394) -> ("ITC Setup"=w392:T11, "Connected"=w393:bool)
                    n352 = local write "ITC Setup"(w392) -> ()
                    n353 = call "ITC503 Get Values.vi"("ITC Setup"=w392) -> ("ITC503 Current Values"=w391:T1)  [unwired: 1 in, 1 out]
                    n354 = Unbundle By Name(w391) -> ("ITC503 Setpoint"=w388:dbl)
                    n355 = Bundle By Name(cluster=T2 {"ITC503 Set Setpoint"=0.0, "ITC503 Set Auto Heater"=TRUE, "ITC503 Set Auto PID"=TRUE, "P"=0.0, "I"=0.0, "D"=0.0} ("ITC503 Settings"), "ITC503 Set Setpoint"=w388) -> (w389:T2)
                    n356 = local write "ITC Settings"(w389) -> ()
                  }
                }
                n357 = case shown="False" w383 {
                  tunnel: [T15."Disabled and Grayed Out" ("Deaktiviert") T15."Enabled" ("Deaktiviert")] -> w382
                  frame False {
                  }
                  frame True {
                  }
                }
                n358 = local write "ITC Status"(w383) -> ()
                n359 = local write "ITC Connect"(w383) -> ()
                n360 = property on="ITC Configure" class="Bool (strict)"("DisabledEnum"=w382) -> ()  [unwired: 2 in, 2 out]
              }
              frame #2 {
                n361 = property on="ITC Running" class="Bool (strict)"("Blinking"=FALSE ("Blinkend")) -> ()  [unwired: 2 in, 2 out]
                n362 = property on="ITC Read" class="Bool (strict)"("Val(Sgnl)"=TRUE ("Wert (signalisierend)")) -> ()  [unwired: 2 in, 2 out]
              }
            }
          }
          event "ITC Read": Value Change {
            n363 = event-data() -> ("Time"=w398:u32, "NewVal"=w401:bool)  [unwired: 1 in, 3 out]
            n364 = local read "ITC Status"() -> (w400:bool)
            n365 = And(x=w400, y=w401) -> (x .and. y?=w399:bool)
            n366 = case shown="True" w399 {
              tunnel: w398 -> [_ w405]
              tunnel: [u32 0 w404] -> w397
              frame False {
                n367 = property on="ITC Running" class="Bool (strict)"("BoolText.Text"="" ("Boolescher Text.Text")) -> ()  [unwired: 2 in, 2 out]
              }
              frame True {
                n368 = stacked-sequence {
                  seq-local: [_ w411 _ _] -> [_ _ w432 _]
                  seq-local: [w406 _ _ _] -> [_ _ _ w440]
                  tunnel: w405 -> [_ w412 _ _]
                  tunnel: [_ _ _ w441] -> w404
                  frame #0 {
                    n369 = Tick Count (ms)() -> (millisecond timer value=w406:u32)
                  }
                  frame #1 {
                    n370 = local read "ITC Setup"() -> (w417:T11)
                    n371 = local read "ITC Gradient Time"() -> (w416:i64)
                    n372 = call "ITC503 Get Values.vi"("ITC Setup"=w417) -> ("ITC503 Current Values"=w411:T1)  [unwired: 1 in, 1 out]
                    n373 = local read "ITC Temp Storage"() -> (w410:dbl)
                    n374 = Unbundle By Name(w411) -> ("ITC503 Temperature"=w409:dbl)
                    n375 = Subtract(x=w412, y=w416) -> (x-y=w415:i64)
                    n376 = Divide(x=w415, y=i64 1000) -> (x/y=w413:dbl)
                    n377 = Equal To 0?(x=w409) -> (x = 0?=w408:bool)
                    n378 = case shown="False" w408 {
                      tunnel: w413 -> [w423 _]
                      tunnel: w411 -> [w422 _]
                      tunnel: w410 -> [w421 _]
                      tunnel: w409 -> [w419 _]
                      frame False {
                        n379 = Subtract(x=w419, y=w421) -> (x-y=w420:dbl)
                        n380 = Divide(x=w420, y=w423) -> (x/y=w424:dbl)
                        n381 = Bundle By Name(cluster=w422, "ITC503 Gradient"=w424) -> (w418:T1)
                        n382 = local write "ITC Current Values"(w418) -> ()
                        n383 = global write "Global Variables.vi" "Global ITC Values"(w418) -> ()
                      }
                      frame True {
                      }
                    }
                    n384 = Not(x=w408) -> (.not. x?=w407:bool)
                    n385 = local write "ITC Status"(w407) -> ()
                  }
                  frame #2 {
                    n386 = Unbundle By Name(w432) -> ("ITC503 Temperature"=w427:dbl, "ITC503 Setpoint"=w433:dbl)
                    n387 = Subtract(x=w427, y=w433) -> (x-y=w434:dbl)
                    n388 = Number To Fractional String(number=w427, precision (6)=i16 2 ("Genauigkeit (6)")) -> (F-format string=w430:string)  [unwired: 2 in]
                    n389 = local write "ITC Temp Storage"(w427) -> ()
                    n390 = Absolute Value(x=w434) -> (abs(x)=w435:dbl)
                    n391 = String Subset(string=w430, length (rest)=5 ("Länge (Rest)")) -> (substring=w428:string)  [unwired: 1 in]
                    n392 = Less?(x=w435, y=2.0) -> (x < y?=w426:bool)
                    n393 = case shown="True" w426 {
                      tunnel: [u32 16711680 u32 0] -> w425
                      frame False {
                      }
                      frame True {
                      }
                    }
                    n394 = property on="ITC Running" class="Bool (strict)"("Value"=w426, "BoolText.Text"=w428, "BoolText.TextColor"=w425) -> ()  [unwired: 2 in, 2 out]
                  }
                  frame #3 {
                    n395 = Tick Count (ms)() -> (millisecond timer value=w439:u32)
                    n396 = local write "ITC Gradient Time"(w439) -> ()
                    n397 = Subtract(x=w439, y=w440) -> (x-y=w441:u32)
                  }
                }
              }
            }
            n398 = local write "ITC Timing"(w397) -> ()
          }
          event "ITC Configure": Value Change {
            n399 = event-data() -> ("NewVal"=w442:bool)  [unwired: 1 in, 4 out]
            n400 = stacked-sequence {
              tunnel: w442 -> [_ w444 _]
              frame #0 {
                n401 = property on="ITC Running" class="Bool (strict)"("Blinking"=TRUE ("Blinkend")) -> ()  [unwired: 2 in, 2 out]
              }
              frame #1 {
                n402 = local read "ITC Status"() -> (w446:bool)
                n403 = And(x=w446, y=w444) -> (x .and. y?=w445:bool)
                n404 = case shown="True" w445 {
                  frame False {
                  }
                  frame True {
                    n405 = local read "ITC Settings"() -> (w447:T2)
                    n406 = local read "ITC Setup"() -> (w448:T11)
                    n407 = call "ITC503 Set Values.vi"("Set Channel"=i16 1, "ITC503 Settings"=w447, "ITC Setup"=w448) -> ()  [unwired: 2 in]
                  }
                }
              }
              frame #2 {
                w451 = FALSE ("Blinkend")
                n408 = property on="ITC Running" class="Bool (strict)"("Blinking"=w451) -> ()  [unwired: 2 in, 2 out]
                n409 = local write "ITC Configure"(w451) -> ()
                n410 = property on="ITC Read" class="Bool (strict)"("Val(Sgnl)"=TRUE ("Wert (signalisierend)")) -> ()  [unwired: 2 in, 2 out]
              }
            }
          }
          event "Drive Connect": Value Change {
            n411 = event-data() -> ("NewVal"=w452:bool)  [unwired: 1 in, 4 out]
            n412 = stacked-sequence {
              tunnel: w452 -> [_ w455 _ _]
              frame #0 {
                n413 = property on="Drive Running" class="Bool (strict)"("Blinking"=TRUE ("Blinkend")) -> ()  [unwired: 2 in, 2 out]
              }
              frame #1 {
                n414 = local read "Drive Connection"() -> (w456:refnum<visa-resource-name>)
                n415 = case shown="True" w455 {
                  tunnel: w456 -> [w461 w463]
                  tunnel: [TRUE ("Success") w462] -> w454
                  frame False {
                    n416 = call "NPC3SG Close.vi"("Drive Visa Name"=w461) -> ()  [unwired: 4 in]
                  }
                  frame True {
                    n417 = call "NPC3SG Connect v10.6.0.vi"("Drive Port"=w463) -> ("Success"=w462:bool)  [unwired: 2 in, 1 out]
                  }
                }
                n418 = Not(x=w455) -> (.not. x?=w458:bool)
                n419 = Exclusive Or(1:w458, 2:w454) -> (0:w459:bool)
                n420 = local write "Drive Connect"(w459) -> ()
                n421 = local write "Drive Status"(w459) -> ()
                n422 = case shown="False" w459 {
                  tunnel: [T15."Disabled and Grayed Out" ("Deaktiviert") T15."Enabled" ("Deaktiviert")] -> w457
                  frame False {
                  }
                  frame True {
                  }
                }
                n423 = property on="Drive Live Controls" class="Clust (strict)"("DisabledEnum"=w457) -> ()  [unwired: 2 in, 2 out]
                n424 = property on="Drive GoTo" class="Bool (strict)"("DisabledEnum"=w457) -> ()  [unwired: 2 in, 2 out]
              }
              frame #2 {
                # "prepare mirroring values to target controls"
                n425 = local write "Drive Copy Target"(TRUE ("Copy Drive Target")) -> ()
              }
              frame #3 {
                n426 = property on="Drive Running" class="Bool (strict)"("Blinking"=FALSE ("Blinkend")) -> ()  [unwired: 2 in, 2 out]
                n427 = property on="Drive Read" class="Bool (strict)"("Val(Sgnl)"=TRUE ("Wert (signalisierend)")) -> ()  [unwired: 2 in, 2 out]
              }
            }
          }
          event "Drive Read": Value Change {
            n428 = event-data() -> ("NewVal"=w472:bool)  [unwired: 1 in, 4 out]
            n429 = local read "Drive Status"() -> (w471:bool)
            n430 = And(x=w471, y=w472) -> (x .and. y?=w470:bool)
            n431 = case shown="True" w470 {
              tunnel: [u32 0 w474] -> w469
              frame False {
              }
              frame True {
                n432 = stacked-sequence {
                  seq-local: [w475 _ _ _] -> [_ _ _ w481]
                  tunnel: [_ _ _ w480] -> w474
                  frame #0 {
                    n433 = Tick Count (ms)() -> (millisecond timer value=w475:u32)
                  }
                  frame #1 {
                    n434 = local read "Drive Connection"() -> (w477:refnum<visa-resource-name>)
                    n435 = call "NPC3SG Get Values.vi"("Drive Visa Name"=w477) -> ("Drive Current Values"=w476:T3)
                    n436 = local write "Drive Live Current Values"(w476) -> ()
                    n437 = local write "Drive Current Values"(w476) -> ()
                    n438 = global write "Global Variables.vi" "Global Piezo Position"(w476) -> ()
                  }
                  frame #2 {
                    n439 = local read "Drive Copy Target"() -> (w478:bool)
                    n440 = case shown="False" w478 {
                      frame False {
                      }
                      frame True {
                        n441 = property on="Drive Copy Target" class="Bool (strict)"("Val(Sgnl)"=TRUE ("Value (Signaling)")) -> ()  [unwired: 2 in, 2 out]
                      }
                    }
                  }
                  frame #3 {
                    n442 = Tick Count (ms)() -> (millisecond timer value=w482:u32)
                    n443 = Subtract(x=w482, y=w481) -> (x-y=w480:u32)
                  }
                }
              }
            }
            "Drive Timing" <- w469
          }
          event "Drive GoTo": Value Change {
            n444 = event-data() -> ("NewVal"=w483:bool)  [unwired: 1 in, 4 out]
            n445 = stacked-sequence {
              tunnel: w483 -> [_ w485 _]
              frame #0 {
                n446 = property on="Drive Running" class="Bool (strict)"("Blinking"=TRUE ("Blinkend")) -> ()  [unwired: 2 in, 2 out]
              }
              frame #1 {
                n447 = local read "Drive Status"() -> (w487:bool)
                n448 = And(x=w487, y=w485) -> (x .and. y?=w486:bool)
                n449 = case shown="True" w486 {
                  frame False {
                  }
                  frame True {
                    n450 = local read "Drive New Positions"() -> (w489:T6)
                    n451 = local read "Drive Connection"() -> (w488:refnum<visa-resource-name>)
                    n452 = control-ref of="Drive Running"() -> (w490:refnum<vi>)
                    n453 = call "NPC3SG Move Absolute.vi"("Running"=w490, "Drive New Abs. Positions"=w489, "Drive Visa Name"=w488) -> ()  [unwired: 2 in]
                  }
                }
              }
              frame #2 {
                w492 = FALSE ("Blinkend")
                n454 = local write "Drive GoTo"(w492) -> ()
                n455 = property on="Drive Running" class="Bool (strict)"("Blinking"=w492) -> ()  [unwired: 2 in, 2 out]
                n456 = property on="Drive Read" class="Bool (strict)"("Val(Sgnl)"=TRUE ("Wert (signalisierend)")) -> ()  [unwired: 2 in, 2 out]
              }
            }
          }
          event Value Change {
            n457 = event-data() -> ("NewVal"=w494:bool)  [unwired: 1 in, 4 out]
            n458 = local read "Drive Status"() -> (w495:bool)
            n459 = And(x=w495, y=w494) -> (x .and. y?=w493:bool)
            n460 = case shown="True" w493 {
              frame False {
              }
              frame True {
                n461 = stacked-sequence {
                  seq-local: [w496 _ _] -> [_ _ _]
                  frame #0 {
                    # "Move and Read"
                    n462 = flat-sequence {
                      tunnel: [w503] -> w499
                      tunnel: [w501] -> w498
                      tunnel: w499 -> [w505]
                      tunnel: w498 -> [w506]
                      tunnel: [w504] -> w497
                      tunnel: w497 -> [w511]
                      tunnel: [w511] -> w496
                      frame #0 {
                        n463 = local read "Drive Live Controls"() -> (w501:T7)
                        n464 = local read "Drive Connection"() -> (w500:refnum<visa-resource-name>)
                        n465 = control-ref of="Drive Running"() -> (w502:refnum<vi>)
                        n466 = call "NPC3SG Live Control.vi"("Running"=w502, "Drive Live Controls"=w501, "Drive Visa Name"=w500) -> ("Reset Switches"=w503:bool)  [unwired: 1 in]
                      }
                      frame #1 {
                        n467 = case shown="False" w505 {
                          tunnel: w506 -> [w507 w510]
                          tunnel: [w507 w509] -> w504
                          frame False {
                          }
                          frame True {
                            w508 = FALSE ("Move Out")
                            n468 = Bundle By Name(cluster=w510, "Move Home"=w508, "Move Down"=w508, "Move Up"=w508, "Move Left"=w508, "Move Right"=w508, "Move Out"=w508, "Move In"=w508) -> (w509:T7)
                          }
                        }
                      }
                      frame #2 {
                        n469 = local write "Drive Live Controls"(w511) -> ()
                      }
                    }
                  }
                  frame #1 {
                    n470 = local write "Drive Copy Target"(TRUE ("Copy Drive Target")) -> ()
                  }
                  frame #2 {
                    n471 = property on="Drive Read" class="Bool (strict)"("Val(Sgnl)"=TRUE ("Wert (signalisierend)")) -> ()  [unwired: 2 in, 2 out]
                  }
                }
              }
            }
          }
          event "Drive Copy Target": Value Change {
            # "this event is triggered after drive readout\nit should usually not be triggered directly by signaling"
            n472 = event-data() -> ("NewVal"=w514:bool)  [unwired: 1 in, 4 out]
            n473 = case shown="True" w514 {
              frame False {
              }
              frame True {
                n474 = stacked-sequence {
                  frame #0 {
                    n475 = local read "Drive Current Values"() -> (w515:T3)
                    n476 = local write "Drive New Positions"(w515) -> ()
                  }
                  frame #1 {
                    n477 = local write "Drive Copy Target"(FALSE ("Copy Drive Target")) -> ()
                  }
                }
              }
            }
          }
          event "Wavelength Recalculate": Value Change {
            n478 = event-data() -> ("NewVal"=w517:bool)  [unwired: 1 in, 4 out]
            n479 = case shown="False" w517 {
              frame False {
              }
              frame True {
                n480 = local read "Mono Current Values"() -> (w520:T9)
                n481 = local read "CCD Area"() -> (w518:T4)
                n482 = call "iHR550 Convert Axis v10.5.0.vi"("CCD Area Format"=w518, "iHR Current Values"=w520) -> ("Wavelengths (nm)"=w519:dbl[])
                n483 = local write "Wavelengths (nm)"(w519) -> ()
                n484 = global write "Global Variables.vi" "Global Wavelengths (nm)"(w519) -> ()
              }
            }
          }
          event Value Change {
            n485 = event-data() -> ("NewVal"=w522:dbl)  [unwired: 1 in, 4 out]
            n486 = local read "JYCCDLib.IJYCCDReqd"() -> (w521:refnum<k7>)
            n487 = call "Symphony Set Integration Time.vi"("JYCCDLib.IJYCCDReqd"=w521, "Integration (s)"=w522) -> ()  [unwired: 13 in, 1 out]
          }
          event "Spectrum Axis": Value Change {
            w535 = u16 2 items=["Pixel", "Wavelength", "Energy"] ("Spectrum Axis")
            w537 = u16 0 items=["Pixel", "Wavelength", "Energy"] ("Spectrum Axis")
            n488 = event-data() -> ("NewVal"=w533:u16)  [unwired: 1 in, 4 out]
            n489 = Equal?(x=w533, y=w537) -> (x = y?=w536:bool)
            n490 = case shown="True" w536 {
              tunnel: [w555 w557] -> w534
              tunnel: [w554 w556] -> w529
              tunnel: "Pixel" ("X Scale.Name Label.Text") -> [_ w556]
              tunnel: "Wavelength (nm)" ("X Scale.Name Label.Text") -> [w554 _]
              frame False {
                n491 = local read "Spectrum Raw WL"() -> (w555:dbl[][])
              }
              frame True {
                n492 = local read "Spectrum Raw PX"() -> (w557:dbl[][])
              }
            }
            n493 = local read "Spectrum Noise"() -> (w524:i64)
            n494 = Equal?(x=w533, y=w535) -> (x = y?=w532:bool)
            n495 = call "Spectrum Noise Subtraction v10.5.0.vi"("Spectrum Noise"=w524, "Spectrum-Array In"=w534) -> ("Spectrum-Array Out"=w531:dbl[][], "Spectrum-Cluster"=w523:T18)
            n496 = case shown="True" w532 {
              tunnel: w531 -> [_ w545]
              tunnel: [w539 w544] -> w530
              tunnel: w523 -> [w539 w543]
              tunnel: w529 -> [w538 w540]
              tunnel: [w538 w542] -> w526
              tunnel: "Energy (eV)" ("X Scale.Name Label.Text") -> [_ w541]
              tunnel: w524 -> [_ w546]
              frame False {
              }
              frame True {
                # "Jacobian Transformation requires noise subtraction"
                n497 = Greater Than 0?(x=w546) -> (x > 0?=w547:bool)
                n498 = case shown="False" w547 {
                  tunnel: w545 -> [_ w553]
                  tunnel: [w549 w552] -> w544
                  tunnel: w543 -> [w549 _]
                  tunnel: [w548 w551] -> w542
                  tunnel: w541 -> [_ w551]
                  tunnel: w540 -> [w548 _]
                  frame False {
                    w550 = u16 1 items=["Pixel", "Wavelength", "Energy"] ("Spectrum Axis")
                    n499 = call "Display Message to User"() -> ()  [unwired: 10 in, 2 out]
                    n500 = local write "Spectrum Axis"(w550) -> ()
                  }
                  frame True {
                    n501 = call "Spectrum Jacobian Transformation v10.5.0.vi"("Spectrum-Array In"=w553) -> ("Spectrum-Cluster"=w552:T18)  [unwired: 1 in, 1 out]
                  }
                }
              }
            }
            n502 = local write "Spectrum"(w530) -> ()
            n503 = property on="Spectrum" class="XYGraph (strict)"("XScale.NameLbl.Text"=w526) -> ()  [unwired: 2 in, 2 out]
          }
          event "Spectrum Noise": Value Change {
            n504 = event-data() -> ("NewVal"=w560:i64)  [unwired: 1 in, 4 out]
            n505 = Greater Than 0?(x=w560) -> (x > 0?=w559:bool)
            n506 = case shown="False" w559 {
              tunnel: [w561 w562] -> w558
              frame False {
                w561 = u16 1 items=["Pixel", "Wavelength", "Energy"] ("Spectrum Axis")
                # "Disable Jacobian Transformation"
              }
              frame True {
                n507 = local read "Spectrum Axis"() -> (w562:u16)
              }
            }
            n508 = property on="Spectrum Axis" class="Ring (strict)"("Val(Sgnl)"=w558) -> ()  [unwired: 2 in, 2 out]
          }
          event "Spectrum Save": Value Change {
            n509 = event-data() -> ("NewVal"=w563:bool)  [unwired: 1 in, 4 out]
            n510 = stacked-sequence {
              tunnel: w563 -> [w564 _]
              frame #0 {
                n511 = case shown="True" w564 {
                  frame False {
                  }
                  frame True {
                    n512 = local read "Mono Current Values"() -> (w567:T9)
                    n513 = local read "Drive Current Values"() -> (w565:T3)
                    n514 = local read "ITC Current Values"() -> (w568:T1)
                    n515 = local read "Spectrum Settings"() -> (w566:T5)
                    n516 = local read "CCD Temperature"() -> (w573:dbl)
                    n517 = local read "CCD Area"() -> (w570:T4)
                    n518 = local read "CCD ADC"() -> (w572:u16)
                    n519 = local read "CCD Gain"() -> (w571:u16)
                    n520 = local read "Image Mode"() -> (w579:bool)
                    n521 = call "Export_fileName v10.6.0.vi"("ITC503 Current Values"=w568, "iHR Current Values"=w567, "Spectra Settings"=w566, "Drive Current Values"=w565) -> ("Filename"=w569:string)  [unwired: 1 in]
                    n522 = case shown="True" w579 {
                      tunnel: [w580 w584] -> w577
                      tunnel: ["Spectrum" ("Export Type") "Image" ("Export Type")] -> w576
                      tunnel: [w581 w588] -> w574
                      tunnel: w570 -> [_ w583]
                      tunnel: w569 -> [w580 w586]
                      frame False {
                        n523 = local read "Spectrum Raw WL"() -> (w581:dbl[][])
                      }
                      frame True {
                        n524 = local read "Image Raw"() -> (w587:i32[][])
                        n525 = Concatenate Strings(w586, "_img" ("string")) -> (w584:string)
                        n526 = call "Image Merge Axes v10.5.1.vi"("Image In"=w587, "CCD Area Format"=w583) -> ("Image Out"=w588:dbl[][])  [unwired: 13 in]
                      }
                    }
                    n527 = local read "Spectrum Autosave"() -> (w575:bool)
                    n528 = local read "Auto Folder"() -> (w578:path)
                    n529 = call "Export_2DtoTxt v10.6.0.vi"("ITC503 Current Values"=w568, "iHR Current Values"=w567, "CCD Temperature"=w573, "CCD Area"=w570, "CCD ADC"=w572, "CCD Gain"=w571, "Auto?"=w575, "Export Type"=w576, "Spectra Settings"=w566, "Filename"=w577, "Data (2D)"=w574, "Auto Folder"=w578) -> ()  [unwired: 7 in, 1 out]
                  }
                }
              }
              frame #1 {
                n530 = local write "Spectrum Save"(FALSE ("Spectrum Save")) -> ()
              }
            }
          }
          event "Spectrum Load": Value Change {
            n531 = event-data() -> ("NewVal"=w591:bool)  [unwired: 1 in, 4 out]
            n532 = case shown="True" w591 {
              frame False {
              }
              frame True {
                n533 = stacked-sequence {
                  seq-local: [w592 _ _] -> [_ w595 _]
                  frame #0 {
                    n534 = call "Load Spectrum.vi"() -> ("Intensity"=w592:dbl[], "Wavelength"=w594:dbl[])  [unwired: 3 in, 1 out]
                    n535 = Build Array(w594, w592) -> (w593:dbl[][])
                    n536 = local write "Spectrum Raw WL"(w593) -> ()
                  }
                  frame #1 {
                    n537 = call <vilib>:"Median.vi"("X"=w595) -> ("median"=w597:dbl)  [unwired: 1 out]
                    n538 = To Long Integer(number=w597) -> (32bit integer=w596:i32)
                    n539 = property on="Spectrum Noise" class="DigNum (strict)"("Val(Sgnl)"=w596) -> ()  [unwired: 2 in, 2 out]
                  }
                  frame #2 {
                    n540 = local write "Spectrum Load"(FALSE ("Spectrum Load")) -> ()
                  }
                }
              }
            }
          }
          event "Spectrum Autosave": Value Change {
            n541 = event-data() -> ("NewVal"=w600:bool)  [unwired: 1 in, 4 out]
            n542 = case shown="False" w600 {
              tunnel: [path "" w606] -> w599
              frame False {
              }
              frame True {
                n543 = call "File Dialog"("prompt"="Choose Save Folder") -> ("selected path"=w608:path, "cancelled"=w602:bool, "error out"=w604:errorcluster)  [unwired: 11 in, 1 out]
                n544 = call <vilib>:"Simple Error Handler.vi"("error in (no error)"=w604) -> ("error?"=w603:bool)  [unwired: 4 in, 4 out]
                n545 = Or(x=w602, y=w603) -> (x .or. y?=w605:bool)
                n546 = case shown="True" w605 {
                  tunnel: w608 -> [w609 _]
                  tunnel: [w609 path ""] -> w606
                  frame False {
                  }
                  frame True {
                    n547 = local write "Spectrum Autosave"(FALSE ("Spectrum Autosave")) -> ()
                  }
                }
              }
            }
            n548 = local write "Auto Folder"(w599) -> ()
          }
          event "Spectrum Maximize": Value Change {
            # "Currently disabled by hiding control!"
            n549 = event-data() -> ("NewVal"=w612:bool)  [unwired: 1 in, 4 out]
            n550 = case shown="False" w612 {
              frame False {
                n551 = local read "Spectrum Properties"() -> (w615:cluster{"Position":T10, "Plot Area Size":T10})
                n552 = Unbundle(w615) -> ("Position"=w614:T10, "Plot Area Size"=w613:T10)
                n553 = stacked-sequence {
                  tunnel: w614 -> [_ w617]
                  tunnel: w613 -> [w616 _]
                  frame #0 {
                    n554 = property on="Spectrum" class="XYGraph (strict)"("Plot Area Size"=w616) -> ()  [unwired: 2 in, 2 out]
                  }
                  frame #1 {
                    n555 = property on="Spectrum" class="XYGraph (strict)"("Position"=w617) -> ()  [unwired: 2 in, 2 out]
                  }
                }
              }
              frame True {
                n556 = property on="Spectrum" class="XYGraph (strict)"() -> ("Bounds"=w638:T10, "Plot Area Size"=w637:T10, "Position"=w635:T19)  [unwired: 2 in, 2 out]
                n557 = Bundle("Position"=w635, "Plot Area Size"=w637) -> (w636:cluster{"Position":T19, "Plot Area Size":T10})  [unwired: 1 in]
                n558 = Unbundle By Name(w638) -> ("Width"=w642:u32, "Height"=w643:u32)
                n559 = Unbundle By Name(w637) -> ("Width"=w645:u32, "Height"=w644:u32)
                n560 = property on="Register" class="TabCtl (strict)"() -> ("Bounds"=w641:T10, "Position"=w630:T19, "Width"=w621:u32, "Height"=w620:u32)  [unwired: 2 in, 2 out]
                n561 = local write "Spectrum Properties"(w636) -> ()
                n562 = Subtract(x=w642, y=w645) -> (x-y=w634:u32)
                n563 = Subtract(x=w643, y=w644) -> (x-y=w631:u32)
                n564 = Add(x=w634, y=u32 25) -> (x+y=w633:u32)
                n565 = Add(x=w631, y=u32 70) -> (x+y=w632:u32)
                n566 = Subtract(x=w621, y=w633) -> (x-y=w640:u32)
                n567 = Subtract(x=w620, y=w632) -> (x-y=w639:u32)
                n568 = Bundle By Name(cluster=w641, "Width"=w640, "Height"=w639) -> (w618:T10)
                n569 = Unbundle By Name(w630) -> ("Left"=w629:i32, "Top"=w626:i32)
                n570 = Add(x=w629, y=20) -> (x+y=w628:i32)
                n571 = Add(x=w626, y=50) -> (x+y=w627:i32)
                n572 = Bundle By Name(cluster=w630, "Left"=w628, "Top"=w627) -> (w619:T19)
                n573 = stacked-sequence {
                  tunnel: w619 -> [w646 _]
                  tunnel: w618 -> [_ w647]
                  frame #0 {
                    n574 = property on="Spectrum" class="XYGraph (strict)"("Position"=w646) -> ()  [unwired: 2 in, 2 out]
                  }
                  frame #1 {
                    n575 = property on="Spectrum" class="XYGraph (strict)"("Plot Area Size"=w647) -> ()  [unwired: 2 in, 2 out]
                  }
                }
              }
            }
          }
          event "Mapping Start": Value Change {
            n576 = event-data() -> ("NewVal"=w648:bool)  [unwired: 1 in, 4 out]
            n577 = case shown="True" w648 {
              frame False {
              }
              frame True {
                n578 = stacked-sequence {
                  frame #0 {
                    # "Make sure we do not try mapping in the image mode."
                    n579 = flat-sequence {
                      frame #0 {
                        n580 = property on="Image Mode" class="Bool (strict)"("Val(Sgnl)"=FALSE ("Value (Signaling)")) -> ()  [unwired: 2 in, 2 out]
                      }
                      frame #1 {
                        n581 = property on="CCD Configure" class="Bool (strict)"("Val(Sgnl)"=TRUE ("Value (Signaling)")) -> ()  [unwired: 2 in, 2 out]
                      }
                    }
                  }
                  frame #1 {
                    n582 = local read "JYCCDLib.IJYCCDReqd"() -> (w689:refnum<k7>)
                    n583 = local read "Drive Current Values"() -> (w684:T3)
                    n584 = local read "ITC Current Values"() -> (w686:T1)
                    n585 = local read "Mono Current Values"() -> (w685:T9)
                    n586 = local read "CCD Temperature"() -> (w691:dbl)
                    n587 = vi-ref "Mapping v10.6.0.vi"() -> (w672:refnum<vi>)
                    n588 = local read "Wavelengths (nm)"() -> (w687:dbl[])
                    n589 = local read "Drive Status"() -> (w683:bool)
                    n590 = local read "Drive Connection"() -> (w688:refnum<visa-resource-name>)
                    n591 = local read "Spectrum Settings"() -> (w690:T5)
                    n592 = local read "CCD Status"() -> (w681:bool)
                    n593 = local read "CCD ADC"() -> (w652:u16)
                    n594 = local read "CCD Area"() -> (w654:T4)
                    n595 = local read "CCD Gain"() -> (w653:u16)
                    n596 = local read "CCD Status"() -> (w665:bool)
                    n597 = Not(x=w683) -> (.not. x?=w682:bool)
                    n598 = Not(x=w681) -> (.not. x?=w680:bool)
                    n599 = Not(x=w665) -> (.not. x?=w664:bool)
                    n600 = Bundle By Name(cluster=T17 {"Drive Connection Port"="", "ITC503 Current Values"={"ITC503 Heater"=0.0, "ITC503 Temperature"=0.0, "ITC503 P"=0.0, "ITC503 I"=0.0, "ITC503 D"=0.0, "ITC503 Setpoint"=0.0, "ITC503 Gradient"=0.0, "ITC503 Heater Auto"=FALSE, "ITC503 PID Auto"=FALSE}, "Wavelengths (nm)"=[], "Drive Current Values"={"Drive X Position"=0.0, "Drive Y Position"=0.0, "Drive Z Position"=0.0}, "iHR Current Values"={"iHR 550 Front Entrance"=0.0, "iHR550 Side Exit"=0.0, "iHR550 Wavelength"=897.9988, "iHR550 Exit Mirror"=2, "iHR550 Grating"="1", "Grating Index"=1}, "Spectra Settings"={"Integration Time"=1.0, "Repetitions"=1, "Mapping Spectra"=TRUE}, "CCD3500 Temperature"=0.0, "Simulate Drive"=FALSE, "Simulate Spectra"=FALSE, "JYCCDLib.IJYCCDReqd"=refnum, "CCD Area"={"XStart"=1, "YStart"=1, "XStop"=2048, "YStop"=512, "XBin"=1, "YBin"=1}, "CCD Gain"=1, "CCD ADC"=0} ("Input Parameters"), "JYCCDLib.IJYCCDReqd"=w689, "Drive Connection Port"=w688, "ITC503 Current Values"=w686, "Wavelengths (nm)"=w687, "Drive Current Values"=w684, "iHR Current Values"=w685, "Spectra Settings"=w690, "CCD3500 Temperature"=w691, "Simulate Drive"=w682, "Simulate Spectra"=w680, "CCD Area"=w654, "CCD Gain"=w653, "CCD ADC"=w652) -> (w673:T17)
                    n601 = invoke class="VI" method="Ctrl Val.Set"(reference=w672, "Control Name"="Simulate Spectra", "Value"=w664) -> (reference out=w671:refnum<vi>, error out=w666:errorcluster)  [unwired: 2 in, 3 out]
                    n602 = local read "Drive Status"() -> (w663:bool)
                    n603 = Not(x=w663) -> (.not. x?=w662:bool)
                    n604 = invoke class="VI" method="Ctrl Val.Set"(reference=w671, error in=w666, "Control Name"="Simulate Drive", "Value"=w662) -> (reference out=w670:refnum<vi>, error out=w667:errorcluster)  [unwired: 1 in, 3 out]
                    n605 = invoke class="VI" method="Ctrl Val.Set"(reference=w670, error in=w667, "Control Name"="Input Parameters", "Value"=w673) -> (reference out=w660:refnum<vi>, error out=w657:errorcluster)  [unwired: 1 in, 3 out]
                    n606 = property on="Measurement Running" class="Bool (strict)"("Blinking"=TRUE ("Blinkend")) -> ()  [unwired: 2 in, 2 out]
                    n607 = invoke class="VI" method="Ctrl Val.Set"(reference=w660, error in=w657, "Control Name"="AutoClose", "Value"=TRUE ("Blinkend")) -> (reference out=w659:refnum<vi>, error out=w658:errorcluster)  [unwired: 1 in, 3 out]
                    n608 = invoke on="Invoke Node" class="VI" method="FP.Open"(reference=w659, error in=w658, "Activate"=TRUE ("Activate?")) -> (reference out=w675:refnum<vi>, error out=w674:errorcluster)  [unwired: 2 in, 3 out]
                    n609 = invoke on="Invoke Node" class="VI" method="Run VI"(reference=w675, error in=w674, "Wait until done"=FALSE ("Wait Until Done"), "Auto Dispose Ref"=TRUE ("Auto Dispose Reference")) -> ()  [unwired: 1 in, 5 out]
                  }
                }
              }
            }
          }
          event "Video Show": Value Change {
            n610 = event-data() -> ("NewVal"=w692:bool)  [unwired: 1 in, 4 out]
            n611 = case shown="True" w692 {
              frame False {
                n612 = call "Video Toolset Stop.vi"() -> ()  [unwired: 3 in]
              }
              frame True {
                n613 = local read "Snapshot Folder"() -> (w694:path)
                n614 = local read "Camera Name"() -> (w693:string)
                n615 = call "Video Toolset Start.vi"("Snapshot Folder"=w694, "Camera Name"=w693) -> ()  [unwired: 1 in]
              }
            }
          }
        }
      }
    }
    frame #3 {
      # "Close Connections"
      n616 = control-ref of="Dieses VI"() -> (w695:refnum<vi>)
      n617 = invoke class="VI" method="Default Vals.Reinit All"(reference=w695) -> ()  [unwired: 2 in, 3 out]
    }
  }
